vi "Pedestal_viewer (Module).vi"(0 "ACQ full DATA file path":path caption="File path", 5 "ChipID list":u32[](array[numeric]) format="%.0x", 7 "quants events per chip":u32[](array[numeric]), 9 "ID summary":string, 11 "ACQ events fets":u32=80 caption="Acquired events") -> ()   [LabVIEW 2015, in "VIPM2.lvlib"]
doc: "<b>Acquisition Data viewer</b>\nInclou ACQ choose Chip Data_viewer.vi"
uses:
  VIPM2.lvlib
  <vilib>/Analysis/NI_AALBase.lvlib
panel:
  out "Barra Load events":i32(slide) scale=-1.0..3600000.0
  in  "X scale max.":dbl=150.0 min=0.0 max=1e+29 step=10.0
  in  "X scale min.":dbl=80.0 min=0.0 max=1e+29 step=10.0
  in  "Y scale":dbl=100.0 min=5.0 max=1e+29 step=10.0
  in  "Take image button":bool
  in  "Choose Chip button":bool
  in  "Close button":bool
  out "Total number of events":u32 caption="Total number of events\nCentrals + Neighbors"
  out "data time":string
  out "Chip ID":string
  out "Trigger histogram 99":T1(graph)
  out "Trigger histogram 98":T1(graph)
  out "Trigger histogram 97":T1(graph)
  out "Trigger histogram 96":T1(graph)
  out "Trigger histogram 95":T1(graph)
  out "Trigger histogram 94":T1(graph)
  out "Trigger histogram 93":T1(graph)
  out "Trigger histogram 92":T1(graph)
  out "Trigger histogram 91":T1(graph)
  out "Trigger histogram 90":T1(graph)
  out "Trigger histogram 89":T1(graph)
  out "Trigger histogram 88":T1(graph)
  out "Trigger histogram 87":T1(graph)
  out "Trigger histogram 86":T1(graph)
  out "Trigger histogram 85":T1(graph)
  out "Trigger histogram 84":T1(graph)
  out "Trigger histogram 83":T1(graph)
  out "Trigger histogram 82":T1(graph)
  out "Trigger histogram 81":T1(graph)
  out "Trigger histogram 80":T1(graph)
  out "Trigger histogram 79":T1(graph)
  out "Trigger histogram 78":T1(graph)
  out "Trigger histogram 77":T1(graph)
  out "Trigger histogram 76":T1(graph)
  out "Trigger histogram 75":T1(graph)
  out "Trigger histogram 74":T1(graph)
  out "Trigger histogram 73":T1(graph)
  out "Trigger histogram 72":T1(graph)
  out "Trigger histogram 71":T1(graph)
  out "Trigger histogram 70":T1(graph)
  out "Trigger histogram 69":T1(graph)
  out "Trigger histogram 68":T1(graph)
  out "Trigger histogram 67":T1(graph)
  out "Trigger histogram 66":T1(graph)
  out "Trigger histogram 65":T1(graph)
  out "Trigger histogram 64":T1(graph)
  out "Trigger histogram 63":T1(graph)
  out "Trigger histogram 62":T1(graph)
  out "Trigger histogram 61":T1(graph)
  out "Trigger histogram 60":T1(graph)
  out "Trigger histogram 59":T1(graph)
  out "Trigger histogram 58":T1(graph)
  out "Trigger histogram 57":T1(graph)
  out "Trigger histogram 56":T1(graph)
  out "Trigger histogram 55":T1(graph)
  out "Trigger histogram 54":T1(graph)
  out "Trigger histogram 53":T1(graph)
  out "Trigger histogram 52":T1(graph)
  out "Trigger histogram 51":T1(graph)
  out "Trigger histogram 50":T1(graph)
  out "Trigger histogram 49":T1(graph)
  out "Trigger histogram 48":T1(graph)
  out "Trigger histogram 47":T1(graph)
  out "Trigger histogram 46":T1(graph)
  out "Trigger histogram 45":T1(graph)
  out "Trigger histogram 44":T1(graph)
  out "Trigger histogram 43":T1(graph)
  out "Trigger histogram 42":T1(graph)
  out "Trigger histogram 41":T1(graph)
  out "Trigger histogram 40":T1(graph)
  out "Trigger histogram 39":T1(graph)
  out "Trigger histogram 38":T1(graph)
  out "Trigger histogram 37":T1(graph)
  out "Trigger histogram 36":T1(graph)
  out "Trigger histogram 35":T1(graph)
  out "Trigger histogram 34":T1(graph)
  out "Trigger histogram 33":T1(graph)
  out "Trigger histogram 32":T1(graph)
  out "Trigger histogram 31":T1(graph)
  out "Trigger histogram 30":T1(graph)
  out "Trigger histogram 29":T1(graph)
  out "Trigger histogram 28":T1(graph)
  out "Trigger histogram 27":T1(graph)
  out "Trigger histogram 26":T1(graph)
  out "Trigger histogram 25":T1(graph)
  out "Trigger histogram 24":T1(graph)
  out "Trigger histogram 23":T1(graph)
  out "Trigger histogram 22":T1(graph)
  out "Trigger histogram 21":T1(graph)
  out "Trigger histogram 20":T1(graph)
  out "Trigger histogram 19":T1(graph)
  out "Trigger histogram 18":T1(graph)
  out "Trigger histogram 17":T1(graph)
  out "Trigger histogram 16":T1(graph)
  out "Trigger histogram 15":T1(graph)
  out "Trigger histogram 14":T1(graph)
  out "Trigger histogram 13":T1(graph)
  out "Trigger histogram 12":T1(graph)
  out "Trigger histogram 11":T1(graph)
  out "Trigger histogram 10":T1(graph)
  out "Trigger histogram 09":T1(graph)
  out "Trigger histogram 08":T1(graph)
  out "Trigger histogram 07":T1(graph)
  out "Trigger histogram 06":T1(graph)
  out "Trigger histogram 05":T1(graph)
  out "Trigger histogram 04":T1(graph)
  out "Trigger histogram 03":T1(graph)
  out "Trigger histogram 01":T1(graph)
  out "Trigger histogram 00":T1(graph)
  out "Trigger histogram 02":T1(graph)
  out "100px Trigger Data":cluster{"1px Trigger Data":u16[]}[](array[cluster])
  # "99"
  # "98"
  # "97"
  # "96"
  # "95"
  # "94"
  # "93"
  # "92"
  # "91"
  # "90"
  # "89"
  # "88"
  # "87"
  # "86"
  # "85"
  # "84"
  # "83"
  # "82"
  # "81"
  # "80"
  # "79"
  # "78"
  # "77"
  # "76"
  # "75"
  # "74"
  # "73"
  # "72"
  # "71"
  # "70"
  # "69"
  # "68"
  # "67"
  # "66"
  # "65"
  # "64"
  # "63"
  # "62"
  # "61"
  # "60"
  # "59"
  # "58"
  # "57"
  # "56"
  # "55"
  # "54"
  # "53"
  # "52"
  # "51"
  # "50"
  # "49"
  # "48"
  # "47"
  # "46"
  # "45"
  # "44"
  # "43"
  # "42"
  # "41"
  # "40"
  # "39"
  # "38"
  # "37"
  # "36"
  # "35"
  # "34"
  # "33"
  # "32"
  # "31"
  # "30"
  # "29"
  # "28"
  # "27"
  # "26"
  # "25"
  # "24"
  # "23"
  # "22"
  # "21"
  # "20"
  # "19"
  # "18"
  # "17"
  # "16"
  # "15"
  # "14"
  # "13"
  # "12"
  # "11"
  # "10"
  # "09"
  # "08"
  # "07"
  # "06"
  # "05"
  # "04"
  # "03"
  # "01"
  # "00"
  # "02"
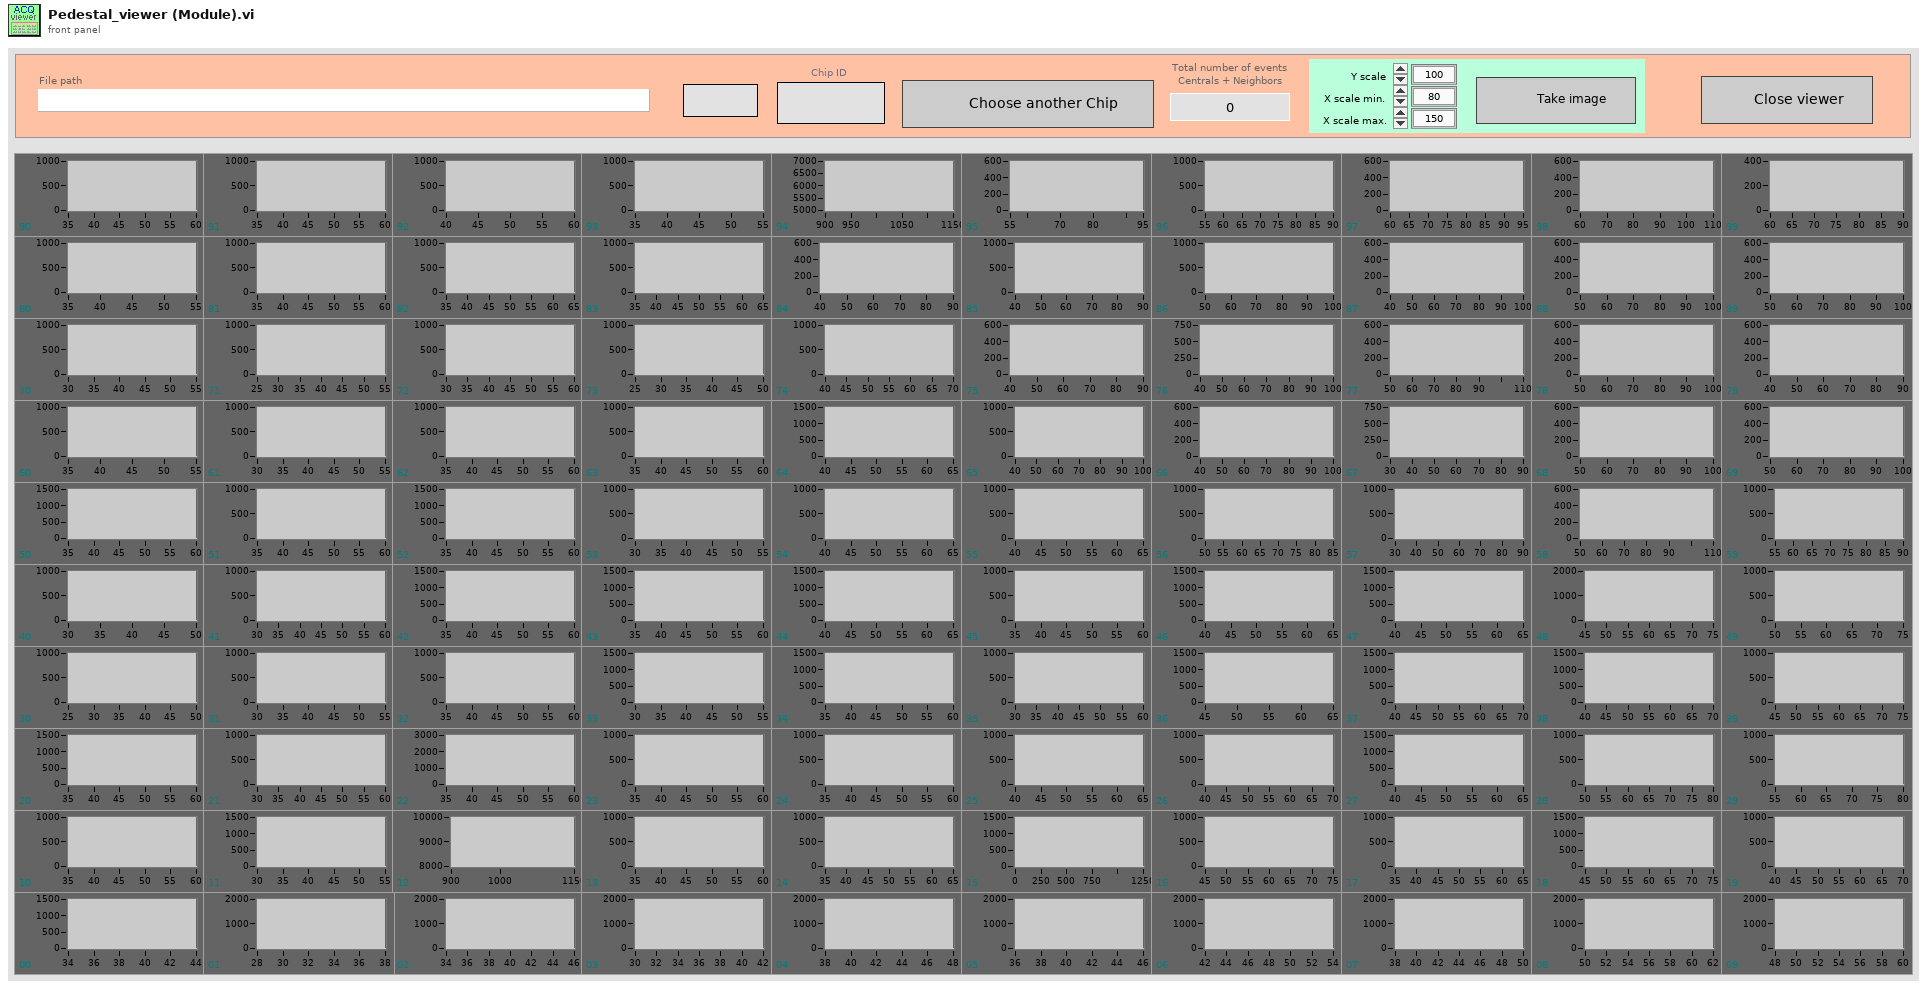
[diagram p1: front panel]
types:
  T1 = cluster{"X Values":dbl[], "Histogram: h(x)":i32[]}
  T2 = enum16{"big-endian, network order", "native, host order", "little-endian"}
  T3 = typedef "imagedata.ctl" = cluster{"image type":i32, "image depth":i32, "image":u8[], "mask":u8[], "colors":u32[], "Rectangle":cluster{"left":i16, "top":i16, "right":i16, "bottom":i16}}
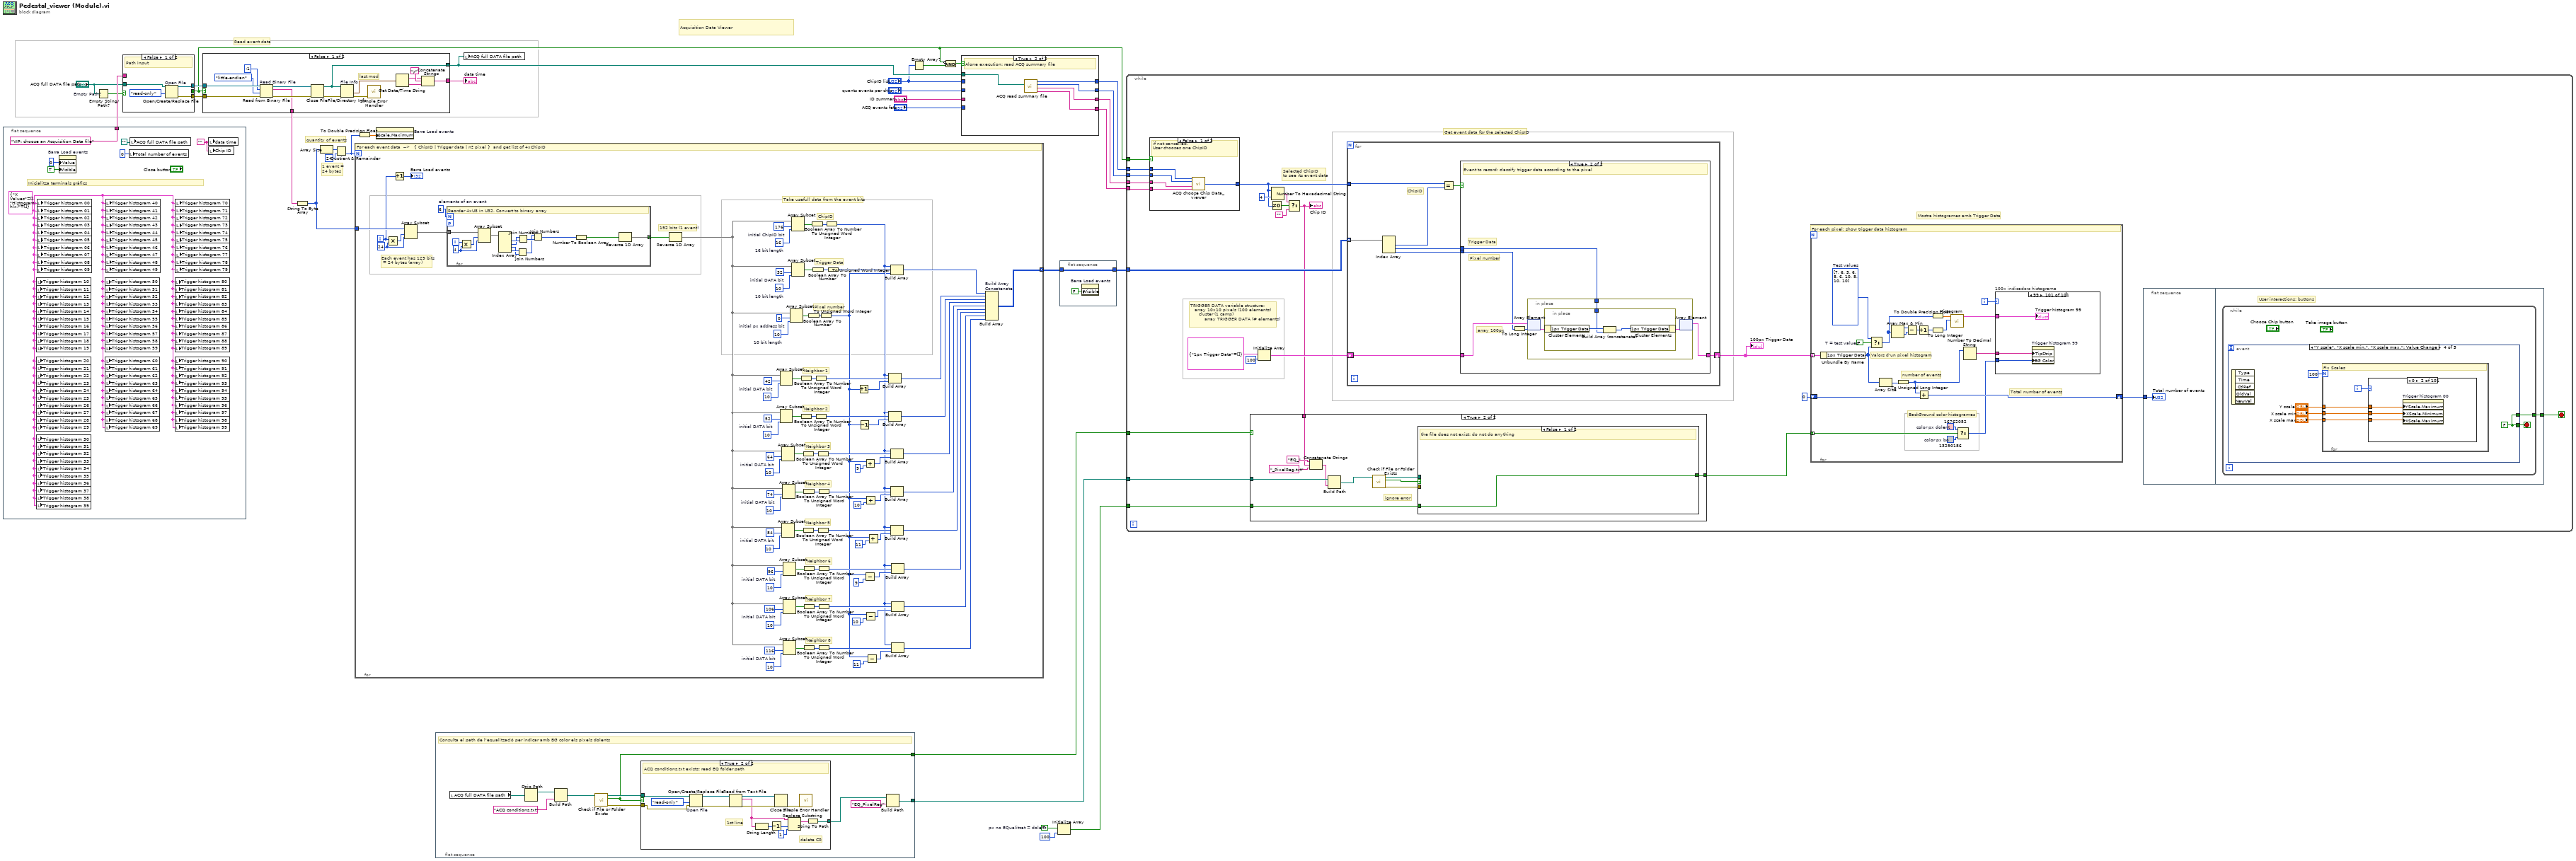
[diagram p0: block diagram]
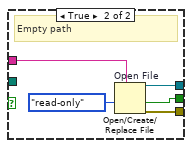
[diagram p3: hidden frame]
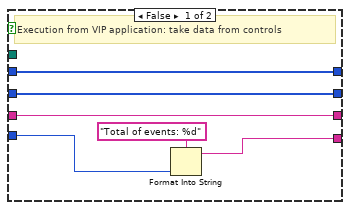
[diagram p5: hidden frame]
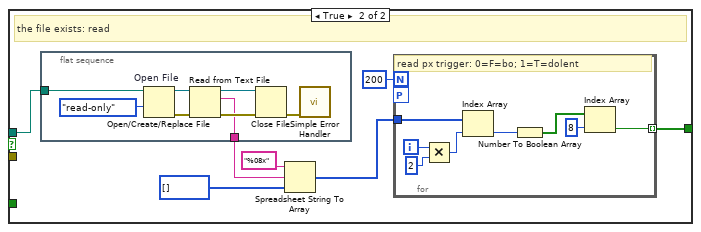
[diagram p7: hidden frame]
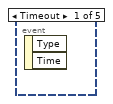
[diagram p9: hidden frame]
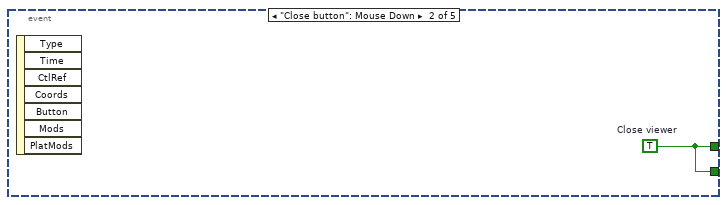
[diagram p10: hidden frame]
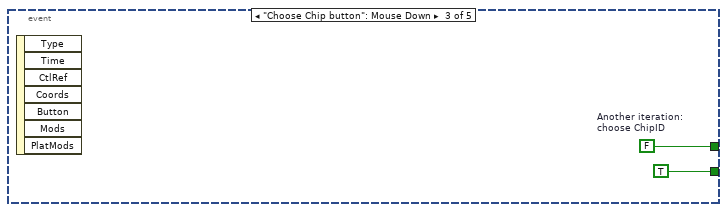
[diagram p11: hidden frame]
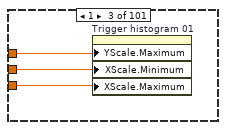
[diagram p13: hidden frame]
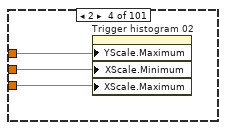
[diagram p14: hidden frame]
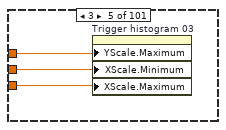
[diagram p15: hidden frame]
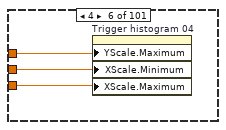
[diagram p16: hidden frame]
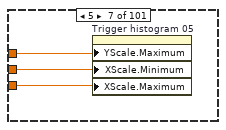
[diagram p17: hidden frame]
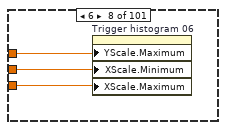
[diagram p18: hidden frame]
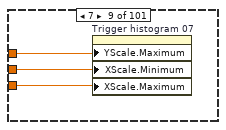
[diagram p19: hidden frame]
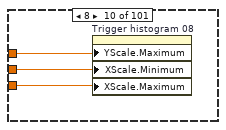
[diagram p20: hidden frame]
diagram:
  w2 = TRUE  # px no EQualitzat = dolent
  # "1 event =\n24 bytes"
  # "quantity of events"
  # "Read event data"
  # "Acquisition Data Viewer"
  n1 = flat-sequence {
    tunnel: ["VIP: choose an Acquisition Data file" ("prompt")] -> w28
    frame #0 {
      w34 = T1 {"X Values"=[], "Histogram: h(x)"=[]} ("Trigger histogram 00")
      w36 = ""
      # "Inicialitza terminals gràfics"
      n2 = local write "Trigger histogram 10"(w34) -> ()
      n3 = local write "Trigger histogram 11"(w34) -> ()
      n4 = local write "Trigger histogram 12"(w34) -> ()
      n5 = local write "Trigger histogram 13"(w34) -> ()
      n6 = local write "Trigger histogram 14"(w34) -> ()
      n7 = local write "Trigger histogram 15"(w34) -> ()
      n8 = local write "Trigger histogram 16"(w34) -> ()
      n9 = local write "Trigger histogram 17"(w34) -> ()
      n10 = local write "Trigger histogram 18"(w34) -> ()
      n11 = local write "Trigger histogram 19"(w34) -> ()
      n12 = local write "Trigger histogram 20"(w34) -> ()
      n13 = local write "Trigger histogram 21"(w34) -> ()
      n14 = local write "Trigger histogram 22"(w34) -> ()
      n15 = local write "Trigger histogram 23"(w34) -> ()
      n16 = local write "Trigger histogram 24"(w34) -> ()
      n17 = local write "Trigger histogram 25"(w34) -> ()
      n18 = local write "Trigger histogram 26"(w34) -> ()
      n19 = local write "Trigger histogram 27"(w34) -> ()
      n20 = local write "Trigger histogram 28"(w34) -> ()
      n21 = local write "Trigger histogram 29"(w34) -> ()
      n22 = local write "Trigger histogram 30"(w34) -> ()
      n23 = local write "Trigger histogram 31"(w34) -> ()
      n24 = local write "Trigger histogram 32"(w34) -> ()
      n25 = local write "Trigger histogram 33"(w34) -> ()
      n26 = local write "Trigger histogram 34"(w34) -> ()
      n27 = local write "Trigger histogram 35"(w34) -> ()
      n28 = local write "Trigger histogram 36"(w34) -> ()
      n29 = local write "Trigger histogram 37"(w34) -> ()
      n30 = local write "Trigger histogram 38"(w34) -> ()
      n31 = local write "Trigger histogram 39"(w34) -> ()
      n32 = local write "Trigger histogram 00"(w34) -> ()
      n33 = local write "Trigger histogram 01"(w34) -> ()
      n34 = local write "Trigger histogram 02"(w34) -> ()
      n35 = local write "Trigger histogram 03"(w34) -> ()
      n36 = local write "Trigger histogram 04"(w34) -> ()
      n37 = local write "Trigger histogram 05"(w34) -> ()
      n38 = local write "Trigger histogram 06"(w34) -> ()
      n39 = local write "Trigger histogram 07"(w34) -> ()
      n40 = local write "Trigger histogram 08"(w34) -> ()
      n41 = local write "Trigger histogram 09"(w34) -> ()
      n42 = property on="Barra Load events" class="Slide (strict)"("Value"=0 ("Barra Load events"), "Visible"=TRUE) -> ()  [unwired: 2 in, 2 out]
      n43 = local write "Trigger histogram 50"(w34) -> ()
      n44 = local write "Trigger histogram 51"(w34) -> ()
      n45 = local write "Trigger histogram 52"(w34) -> ()
      n46 = local write "Trigger histogram 53"(w34) -> ()
      n47 = local write "Trigger histogram 54"(w34) -> ()
      n48 = local write "Trigger histogram 55"(w34) -> ()
      n49 = local write "Trigger histogram 56"(w34) -> ()
      n50 = local write "Trigger histogram 57"(w34) -> ()
      n51 = local write "Trigger histogram 58"(w34) -> ()
      n52 = local write "Trigger histogram 59"(w34) -> ()
      n53 = local write "Trigger histogram 60"(w34) -> ()
      n54 = local write "Trigger histogram 61"(w34) -> ()
      n55 = local write "Trigger histogram 62"(w34) -> ()
      n56 = local write "Trigger histogram 63"(w34) -> ()
      n57 = local write "Trigger histogram 64"(w34) -> ()
      n58 = local write "Trigger histogram 65"(w34) -> ()
      n59 = local write "Trigger histogram 66"(w34) -> ()
      n60 = local write "Trigger histogram 67"(w34) -> ()
      n61 = local write "Trigger histogram 68"(w34) -> ()
      n62 = local write "Trigger histogram 69"(w34) -> ()
      n63 = local write "Trigger histogram 40"(w34) -> ()
      n64 = local write "Trigger histogram 41"(w34) -> ()
      n65 = local write "Trigger histogram 42"(w34) -> ()
      n66 = local write "Trigger histogram 43"(w34) -> ()
      n67 = local write "Trigger histogram 44"(w34) -> ()
      n68 = local write "Trigger histogram 45"(w34) -> ()
      n69 = local write "Trigger histogram 46"(w34) -> ()
      n70 = local write "Trigger histogram 47"(w34) -> ()
      n71 = local write "Trigger histogram 48"(w34) -> ()
      n72 = local write "Trigger histogram 49"(w34) -> ()
      n73 = local write "Total number of events"(u32 0 ("Total number of events")) -> ()
      n74 = local write "ACQ full DATA file path"(path "") -> ()
      n75 = local write "Trigger histogram 80"(w34) -> ()
      n76 = local write "Trigger histogram 81"(w34) -> ()
      n77 = local write "Trigger histogram 82"(w34) -> ()
      n78 = local write "Trigger histogram 83"(w34) -> ()
      n79 = local write "Trigger histogram 84"(w34) -> ()
      n80 = local write "Trigger histogram 85"(w34) -> ()
      n81 = local write "Trigger histogram 86"(w34) -> ()
      n82 = local write "Trigger histogram 87"(w34) -> ()
      n83 = local write "Trigger histogram 88"(w34) -> ()
      n84 = local write "Trigger histogram 89"(w34) -> ()
      n85 = local write "Trigger histogram 90"(w34) -> ()
      n86 = local write "Trigger histogram 91"(w34) -> ()
      n87 = local write "Trigger histogram 92"(w34) -> ()
      n88 = local write "Trigger histogram 93"(w34) -> ()
      n89 = local write "Trigger histogram 94"(w34) -> ()
      n90 = local write "Trigger histogram 95"(w34) -> ()
      n91 = local write "Trigger histogram 96"(w34) -> ()
      n92 = local write "Trigger histogram 97"(w34) -> ()
      n93 = local write "Trigger histogram 98"(w34) -> ()
      n94 = local write "Trigger histogram 99"(w34) -> ()
      n95 = local write "Trigger histogram 70"(w34) -> ()
      n96 = local write "Trigger histogram 71"(w34) -> ()
      n97 = local write "Trigger histogram 72"(w34) -> ()
      n98 = local write "Trigger histogram 73"(w34) -> ()
      n99 = local write "Trigger histogram 74"(w34) -> ()
      n100 = local write "Trigger histogram 75"(w34) -> ()
      n101 = local write "Trigger histogram 76"(w34) -> ()
      n102 = local write "Trigger histogram 77"(w34) -> ()
      n103 = local write "Trigger histogram 78"(w34) -> ()
      n104 = local write "Trigger histogram 79"(w34) -> ()
      n105 = local write "data time"(w36) -> ()
      n106 = local write "Chip ID"(w36) -> ()
    }
  }
  n107 = Empty String/Path? "Empty Path?"(string/path="ACQ full DATA file path") -> (empty?=w27:bool)
  n108 = case shown="False" w27 {
    tunnel: [w41 w46] -> w31
    tunnel: [w40 w45] -> w30
    tunnel: [_ w44] -> w7
    tunnel: w28 -> [_ w43]
    tunnel: "ACQ full DATA file path" -> [w39 _]
    frame False {
      # "Path input"
      n109 = Open/Create/Replace File "Open File"(file path (use dialog)=w39, access (0:read/write)=enum16{"read/write", "read-only", "write-only"}."read-only") -> (refnum out=w40:refnum<file>, error out=w41:errorcluster)  [unwired: 4 in, 1 out]
    }
    frame True {
      # "Empty path"
      n110 = Open/Create/Replace File "Open File"(prompt=w43, access (0:read/write)=enum16{"read/write", "read-only", "write-only"}."read-only") -> (refnum out=w45:refnum<file>, cancelled=w44:bool, error out=w46:errorcluster)  [unwired: 4 in]
    }
  }
  n111 = case shown="False" w7 {
    tunnel: w31 -> [w62 _]
    tunnel: w30 -> [w61 _]
    tunnel: [w56 _] -> w23
    tunnel: [w49 _] -> w29
    tunnel: [w48 _] -> w18
    frame False {
      # "last mod"
      n112 = Read from Binary File "Read Binary File"(8:w62, 9:T2."little-endian" ("byte order (0:big-endian, network order)"), 10:-1 ("count (1)"), 11:w61) -> (0:w59:errorcluster, 2:w56:string, 3:w58:refnum<file>)  [unwired: 2 in, 1 out]
      n113 = Close File(refnum=w58, error in=w59) -> (path=w48:path, error out=w55:errorcluster)
      n114 = File/Directory Info "File Info"(path=w48, error in=w55) -> (last mod=w50:timestamp, error out=w54:errorcluster)  [unwired: 5 out]
      n115 = call <vilib>:"Simple Error Handler.vi"("error in (no error)"=w54) -> ()  [unwired: 4 in, 5 out]
      n116 = Get Date/Time String(seconds (now)=w50) -> (date string=w51:string, time string=w53:string)  [unwired: 2 in]
      n117 = Concatenate Strings(w51, "\r", w53) -> (w49:string)
    }
    frame True {
      # "Openning cancelled"
    }
  }
  "data time" <- w29
  n118 = String To Byte Array(string=w23) -> (unsigned byte array=w6:u8[])
  n119 = Array Size(array=w6) -> (size(s)=w24:i32)
  n120 = Quotient & Remainder(x=w24, y=24) -> (floor(x/y)=w21:i32)  [unwired: 1 out]
  n121 = for {
    N: w21 -> [_]
    tunnel: w6 -> [w146]
    tunnel: [w128] -> w19 mode=concatenating
    i -> [w130]
    w89 = 116  # initial DATA bit
    w94 = 106  # initial DATA bit
    w99 = 96  # initial DATA bit
    w104 = 84  # initial DATA bit
    w109 = 74  # initial DATA bit
    w114 = 64  # initial DATA bit
    w119 = 52  # initial DATA bit
    w126 = 42  # initial DATA bit
    w135 = 10  # 10 bit length
    w136 = 0  # initial px address bit
    w140 = 10  # 10 bit length
    w139 = 32  # initial DATA bit
    w143 = 16  # 16 bit length
    w144 = 176  # initial ChipID bit
    w149 = 24 ("y")
    w150 = 6  # elements of an event
    # "Neighbor 8"
    # "Neighbor 7"
    # "Neighbor 6"
    # "Neighbor 5"
    # "Neighbor 4"
    # "Neighbor 3"
    # "Neighbor 2"
    # "Neighbor 1"
    # "Take usefull data from the event bits"
    # "Pixel number"
    # "Trigger Data"
    # "ChipID"
    # "192 bits (1 event)"
    # "Each event has 129 bits\n = 24 bytes (array)"
    # "For each event data  -->   { ChipID | Trigger data | nº pixel }  and get list of 4xChipID"
    n122 = Multiply(x=w130, y=w149) -> (x*y=w148:i32)
    n123 = Increment(x=w130) -> (x+1=→"Barra Load events":i32)
    n124 = Array Subset "Array Subset"(array=w146, index=w148, length=w149) -> (w147:u8[])
    n125 = for {
      N: w150 -> [_]
      tunnel: w147 -> [w163]
      workers-P: _ -> [_]
      tunnel: [w151] -> w145 mode=concatenating
      i -> [w164]
      w161 = 4 ("y")
      # "Reorder 4xU8 in U32. Convert to binary array"
      n126 = Multiply(x=w164, y=w161) -> (x*y=w162:i32)
      n127 = Array Subset "Array Subset"(array=w163, index=w162, length=w161) -> (w160:u8[])
      n128 = Index Array(array=w160) -> (element #1=w159:u8, element #2=w158:u8, element #3=w156:u8, element #4=w157:u8)  [unwired: 4 in]
      n129 = Join Numbers(hi=w157, lo=w156) -> ((hi.lo)=w154:u16)
      n130 = Join Numbers(hi=w158, lo=w159) -> ((hi.lo)=w155:u16)
      n131 = Join Numbers(hi=w154, lo=w155) -> ((hi.lo)=w152:u32)
      n132 = Number To Boolean Array(number=w152) -> (Boolean array=w153:bool[])
      n133 = Reverse 1D Array(array=w153) -> (reversed array=w151:bool[])
    }
    n134 = Reverse 1D Array(array=w145) -> (reversed array=w68:bool[])
    n135 = Array Subset "Array Subset"(array=w68, index=w126, length=10 ("10 bit length")) -> (w124:bool[])
    n136 = Array Subset "Array Subset"(array=w68, index=w119, length=10 ("10 bit length")) -> (w117:bool[])
    n137 = Array Subset "Array Subset"(array=w68, index=w114, length=10 ("10 bit length")) -> (w112:bool[])
    n138 = Array Subset "Array Subset"(array=w68, index=w104, length=10 ("10 bit length")) -> (w102:bool[])
    n139 = Array Subset "Array Subset"(array=w68, index=w109, length=10 ("10 bit length")) -> (w107:bool[])
    n140 = Array Subset "Array Subset"(array=w68, index=w99, length=10 ("10 bit length")) -> (w97:bool[])
    n141 = Array Subset "Array Subset"(array=w68, index=w94, length=10 ("10 bit length")) -> (w92:bool[])
    n142 = Array Subset "Array Subset"(array=w68, index=w89, length=10 ("10 bit length")) -> (w87:bool[])
    n143 = Array Subset "Array Subset"(array=w68, index=w136, length=w135) -> (w134:bool[])
    n144 = Array Subset "Array Subset"(array=w68, index=w144, length=w143) -> (w142:bool[])
    n145 = Array Subset "Array Subset"(array=w68, index=w139, length=w140) -> (w137:bool[])
    n146 = Boolean Array To Number(Boolean array=w124) -> (number=w125:u32)
    n147 = Boolean Array To Number(Boolean array=w117) -> (number=w118:u32)
    n148 = Boolean Array To Number(Boolean array=w112) -> (number=w113:u32)
    n149 = Boolean Array To Number(Boolean array=w102) -> (number=w103:u32)
    n150 = Boolean Array To Number(Boolean array=w107) -> (number=w108:u32)
    n151 = Boolean Array To Number(Boolean array=w97) -> (number=w98:u32)
    n152 = Boolean Array To Number(Boolean array=w92) -> (number=w93:u32)
    n153 = Boolean Array To Number(Boolean array=w87) -> (number=w88:u32)
    n154 = Boolean Array To Number(Boolean array=w134) -> (number=w133:u32)
    n155 = Boolean Array To Number(Boolean array=w142) -> (number=w141:u32)
    n156 = Boolean Array To Number(Boolean array=w137) -> (number=w138:u32)
    n157 = To Unsigned Word Integer(number=w125) -> (unsigned 16bit integer=w123:u16)
    n158 = To Unsigned Word Integer(number=w118) -> (unsigned 16bit integer=w116:u16)
    n159 = To Unsigned Word Integer(number=w113) -> (unsigned 16bit integer=w111:u16)
    n160 = To Unsigned Word Integer(number=w103) -> (unsigned 16bit integer=w101:u16)
    n161 = To Unsigned Word Integer(number=w108) -> (unsigned 16bit integer=w106:u16)
    n162 = To Unsigned Word Integer(number=w98) -> (unsigned 16bit integer=w96:u16)
    n163 = To Unsigned Word Integer(number=w93) -> (unsigned 16bit integer=w91:u16)
    n164 = To Unsigned Word Integer(number=w88) -> (unsigned 16bit integer=w86:u16)
    n165 = To Unsigned Word Integer(number=w133) -> (unsigned 16bit integer=w66:u16)
    n166 = To Unsigned Word Integer(number=w141) -> (unsigned 16bit integer=w67:u16)
    n167 = To Unsigned Word Integer(number=w138) -> (unsigned 16bit integer=w132:u16)
    n168 = Increment(x=w66) -> (x+1=w122:u16)
    n169 = Decrement(x=w66) -> (x-1=w85:u16)
    n170 = Subtract(x=w66, y=u16 9) -> (x-y=w73:u16)
    n171 = Add(x=w66, y=u16 9) -> (x+y=w82:u16)
    n172 = Add(x=w66, y=u16 10) -> (x+y=w79:u16)
    n173 = Subtract(x=w66, y=u16 10) -> (x-y=w70:u16)
    n174 = Subtract(x=w66, y=u16 11) -> (x-y=w64:u16)
    n175 = Add(x=w66, y=u16 11) -> (x+y=w76:u16)
    n176 = Build Array "Build Array"(w67, w123, w122) -> (w121:u16[])
    n177 = Build Array "Build Array"(w67, w116, w85) -> (w84:u16[])
    n178 = Build Array "Build Array"(w67, w111, w82) -> (w81:u16[])
    n179 = Build Array "Build Array"(w67, w101, w76) -> (w75:u16[])
    n180 = Build Array "Build Array"(w67, w132, w66) -> (w129:u16[])
    n181 = Build Array "Build Array"(w67, w106, w79) -> (w78:u16[])
    n182 = Build Array "Build Array"(w67, w96, w73) -> (w72:u16[])
    n183 = Build Array "Build Array"(w67, w91, w70) -> (w69:u16[])
    n184 = Build Array "Build Array"(w67, w86, w64) -> (w63:u16[])
    n185 = Build Array "Build Array\nConcatenate"(w129, w121, w84, w81, w78, w75, w72, w69, w63) -> (w128:u16[][])
  }
  n186 = To Double Precision Float(number=w21) -> (double precision float=w22:dbl)
  n187 = property on="Barra Load events" class="Slide (strict)"("Scale.Maximum"=w22) -> ()  [unwired: 2 in, 2 out]
  n188 = flat-sequence {
    tunnel: [w165] -> w4
    tunnel: [w168] -> w5
    frame #0 {
      # "Consulta el path de l'equalització per indicar amb BG color els pixels dolents"
      n189 = local read "ACQ full DATA file path"() -> (w169:path)
      n190 = Strip Path(path=w169) -> (stripped path=w170:path)  [unwired: 1 out]
      n191 = Build Path(base path=w170, name or relative path="ACQ conditions.txt") -> (appended path=w172:path)
      n192 = call <vilib>:"Check if File or Folder Exists.vi"("path"=w172) -> ("error out"=w174:errorcluster, "file or folder exists?"=w168:bool, "dup path"=w173:path)  [unwired: 8 in]
      n193 = case shown="True" w168 {
        tunnel: w173 -> [_ w188]
        tunnel: w174 -> [_ w186]
        tunnel: [_ w175] -> w166
        frame False {
          # "ACQ conditions.txt doesn't exist"
        }
        frame True {
          # "delete CR"
          # "1st line"
          # "ACQ conditions.txt exists: read EQ folder path"
          n194 = Open/Create/Replace File "Open File"(file path (use dialog)=w188, error in=w186, access (0:read/write)=enum16{"read/write", "read-only", "write-only"}."read-only") -> (refnum out=w185:refnum<file>, error out=w184:errorcluster)  [unwired: 3 in, 1 out]
          n195 = Read from Text File(file (use dialog)=w185, error in=w184) -> (refnum out=w183:refnum<file>, text=w176:string, error out=w182:errorcluster)  [unwired: 2 in, 1 out]
          n196 = String Length(string=w176) -> (length=w180:i32)
          n197 = Decrement(x=w180) -> (x-1=w179:i32)
          n198 = Close File(refnum=w183, error in=w182) -> (error out=w181:errorcluster)  [unwired: 1 out]
          n199 = Replace Substring(2:1 ("length (len. of substring)"), 3:w179, 5:w176) -> (1:w177:string)  [unwired: 1 in, 1 out]
          n200 = call <vilib>:"Simple Error Handler.vi"("error in (no error)"=w181) -> ()  [unwired: 4 in, 5 out]
          n201 = String To Path(string=w177) -> (path=w175:path)
        }
      }
      n202 = Build Path(base path=w166, name or relative path="EQ_PixelReg") -> (appended path=w165:path)
    }
  }
  n203 = local write "ACQ full DATA file path"(w18) -> ()
  n204 = Empty Array?(array="ChipID list") -> (empty?=w9:bool)
  n205 = Compound Arithmetic op=AND(invert w7, w9) -> (w8:bool)
  n206 = case shown="True" w8 {
    tunnel: w18 -> [_ w199]
    tunnel: "ChipID list" -> [w194 _]
    tunnel: [w194 w198] -> w10
    tunnel: [w193 w197] -> w11
    tunnel: "quants events per chip" -> [w193 _]
    tunnel: "ID summary" -> [w192 _]
    tunnel: "ACQ events fets" -> [w190 _]
    tunnel: [w192 w196] -> w12
    tunnel: [w189 w195] -> w13
    frame False {
      # "Execution from VIP application: take data from controls"
      n207 = Format Into String "Format Into String"(format string="Total of events: %d", w190) -> (resulting string=w189:string)  [unwired: 2 in, 1 out]
    }
    frame True {
      # "Alone execution: read ACQ summary file"
      n208 = call "ACQ read summary file.vi"("ACQ binary data file path"=w199) -> ("Total of events"=w195:string, "ID summary"=w196:string, "quants events per chip"=w197:u32[], "ChipID list"=w198:u32[])  [unwired: 7 in]
    }
  }
  n209 = Initialize Array "Initialize Array"(w2, 100 ("dimension size")) -> (w1:bool[])
  n210 = flat-sequence {
    tunnel: [w201] -> w20
    tunnel: w19 -> [w201]
    frame #0 {
      n211 = property on="Barra Load events" class="Slide (strict)"("Visible"=FALSE) -> ()  [unwired: 2 in, 2 out]
    }
  }
  n212 = while {
    tunnel: w20 -> [w224]
    tunnel: w13 -> [w211]
    tunnel: w12 -> [w210]
    tunnel: w11 -> [w209]
    tunnel: w10 -> [w208]
    tunnel: w7 -> [w207]
    tunnel: w5 -> [w205]
    tunnel: w4 -> [w204]
    tunnel: w1 -> [w203]
    stop <- w218 stop-if-true
    # "Mostra histogrames amb Trigger Data"
    # "TRIGGER DATA variable structure:\n   array 10x10 pixels (100 elements)\n      cluster (1 camp)\n          array TRIGGER DATA (# elements)"
    # "Get event data for the selected ChipID"
    # "Selected ChipID\nto see its event data"
    n213 = case shown="False" w207 {
      tunnel: [w265 _] -> w212
      tunnel: w211 -> [w264 _]
      tunnel: w210 -> [w263 _]
      tunnel: w209 -> [w262 _]
      tunnel: w208 -> [w261 _]
      frame False {
        # "if not cancelled,\nUser chooses one ChipID"
        n214 = call "ACQ choose Chip Data_viewer.vi"("Chip ID list"=w261, "quants events per Chip"=w262, "summary IDs"=w263, "Total of events"=w264) -> ("ChipID choosed"=w265:u16)  [unwired: 11 in]
      }
      frame True {
      }
    }
    n215 = Initialize Array "Initialize Array"(cluster{"1px Trigger Data":u16[]} {"1px Trigger Data"=[]} ("1px Trigger Data"), 100 ("dimension size")) -> (w221:cluster{"1px Trigger Data":u16[]}[])
    n216 = Not Equal To 0?(x=w212) -> (x != 0?=w215:bool)
    n217 = Number To Hexadecimal String(1:i16 4 ("width (-)"), 2:w212) -> (0:w216:string)
    n218 = Select(t=w216, s=w215, f="") -> (s? t:f=w206:string)
    "Chip ID" <- w206
    n219 = case shown="True" w205 {
      tunnel: w204 -> [_ w236]
      tunnel: w206 -> [_ w234]
      tunnel: [w225 w227] -> w202
      tunnel: w203 -> [w225 w226]
      frame False {
      }
      frame True {
        # "ignore error"
        n220 = Concatenate Strings "Concatenate Strings"("EQ_", w234, "_PixelReg.txt") -> (w232:string)
        n221 = Build Path(base path=w236, name or relative path=w232) -> (appended path=w231:path)
        n222 = call <vilib>:"Check if File or Folder Exists.vi"("path"=w231) -> ("error out"=w228:errorcluster, "file or folder exists?"=w229:bool, "dup path"=w230:path)  [unwired: 8 in]
        n223 = case shown="False" w229 {
          tunnel: w230 -> [_ w244]
          tunnel: w228 -> [_ _]
          tunnel: [w237 w238] -> w227
          tunnel: w226 -> [w237 _]
          frame False {
            # "the file does not exist: do not do anything"
          }
          frame True {
            # "the file exists: read"
            n224 = flat-sequence {
              tunnel: w244 -> [w260]
              tunnel: [w253] -> w243
              frame #0 {
                n225 = Open/Create/Replace File "Open File"(file path (use dialog)=w260, access (0:read/write)=enum16{"read/write", "read-only", "write-only"}."read-only") -> (refnum out=w257:refnum<file>, error out=w258:errorcluster)  [unwired: 4 in, 1 out]
                n226 = Read from Text File(file (use dialog)=w257, error in=w258) -> (refnum out=w256:refnum<file>, text=w253:string, error out=w255:errorcluster)  [unwired: 2 in, 1 out]
                n227 = Close File(refnum=w256, error in=w255) -> (error out=w254:errorcluster)  [unwired: 1 out]
                n228 = call <vilib>:"Simple Error Handler.vi"("error in (no error)"=w254) -> ()  [unwired: 4 in, 5 out]
              }
            }
            n229 = Spreadsheet String To Array(format string="%08x", spreadsheet string=w243, array type (2D Dbl)=u32[] []) -> (array=w240:u32[])  [unwired: 1 in]
            n230 = for {
              N: 200 -> [_]
              tunnel: w240 -> [w249]
              tunnel: [w245] -> w238 mode=indexing
              workers-P: _ -> [_]
              i -> [w252]
              # "read px trigger: 0=F=bo; 1=T=dolent"
              n231 = Multiply(x=w252, y=2) -> (x*y=w250:i32)
              n232 = Index Array "Index Array"(array=w249, index=w250) -> (element=w248:u32)
              n233 = Number To Boolean Array(number=w248) -> (Boolean array=w247:bool[])
              n234 = Index Array "Index Array"(array=w247, index=8) -> (element=w245:bool)
            }
          }
        }
      }
    }
    n235 = for {
      tunnel: w224 -> [w921] mode=indexing
      tunnel: w212 -> [w925]
      shift-right: [w922] -> w213
      shift-left: w221 -> [w923]
      # "ChipID"
      n236 = Index Array "Index Array"(array=w921) -> (element #1=w918:u16, element #2=w920:u16, element #3=w919:u16)  [unwired: 3 in]
      n237 = Equal?(x=w925, y=w918) -> (x = y?=w924:bool)
      n238 = case shown="True" w924 {
        tunnel: w923 -> [w926 w931]
        tunnel: [w926 w930] -> w922
        tunnel: w920 -> [_ w929]
        tunnel: w919 -> [_ w927]
        frame False {
          # "This event is not from selected ChipID: skip"
        }
        frame True {
          # "array 100px"
          # "Pixel number"
          # "Trigger Data"
          # "Event to record: classify trigger data according to the pixel"
          n239 = To Long Integer(number=w927) -> (32bit integer=w928:i32)
          n240 = in-place {
            in-place-border: w929 -> [w932]
            n241 = in-place-array #1(w931, w928) -> (w934:cluster{"1px Trigger Data":u16[]})
            n242 = in-place {
              in-place-border: w932 -> [w936]
              n243 = in-place-cluster #2(w934) -> ("1px Trigger Data"=w937:u16[])
              n244 = Build Array (concatenate) "Build Array"(w937, w936) -> (w935:u16[])
              n245 = in-place-cluster #2("1px Trigger Data"=w935) -> (w933:cluster{"1px Trigger Data":u16[]})
            }
            n246 = in-place-array #1(w933) -> (w930:cluster{"1px Trigger Data":u16[]}[])  [unwired: 1 out]
          }
        }
      }
    }
    "100px Trigger Data" <- w213
    n247 = for {
      tunnel: w213 -> [w611] mode=indexing
      shift-right: [w604] -> w219
      shift-left: u32 0 -> [w603]
      tunnel: w202 -> [w596] mode=indexing
      i -> [w610]
      w599 = u32 13290186  # color px bo
      w598 = u32 16762052  # color px dolent
      w607 = u16[] [7, 6, 5, 6, 8, 6, 10, 8, 10, 10]  # Test values
      w606 = FALSE  # T = test values
      # "BackGround color histogrames"
      # "Total number of events"
      # "number of events"
      # "Valors d'un pixel histogram"
      # "For each pixel: show trigger data histogram"
      n248 = Unbundle By Name(w611) -> ("1px Trigger Data"=w605:u16[])
      n249 = Select(t=w607, s=w606, f=w605) -> (s? t:f=w608:u16[])
      n250 = Array Size(array=w605) -> (size(s)=w602:i32)
      n251 = Array Max & Min(array=w608) -> (max value=w614:u16, min value=w613:u16)  [unwired: 2 out]
      n252 = To Unsigned Long Integer(number=w602) -> (unsigned 32bit integer=w601:u32)
      n253 = Subtract(x=w614, y=w613) -> (x-y=w612:u16)
      n254 = Increment(x=w612) -> (x+1=w616:u16)
      n255 = Add(x=w601, y=w603) -> (x+y=w604:u32)
      n256 = To Long Integer(number=w616) -> (32bit integer=w617:i32)
      n257 = To Double Precision Float(number=w608) -> (double precision float=w615:dbl[])
      n258 = call <vilib>:"Histogram.vi"("intervals"=w617, "X"=w615) -> ("Histogram Graph"=w609:T1)  [unwired: 6 in, 3 out]
      n259 = Select(t=w598, s=w596, f=w599) -> (s? t:f=w597:u32)
      n260 = Number To Decimal String(number=w601) -> (decimal integer string=w600:string)  [unwired: 1 in]
      n261 = case "100x indicadors histograma" shown="99" w610 {
        tunnel: w609 -> [_ w620 w623 w626 w629 w632 w635 w638 w641 w644 w647 w650 w653 w656 w659 w662 w665 w668 w671 w674 w677 w680 w683 w686 w689 w692 w695 w698 w701 w704 w707 w710 w713 w716 w719 w722 w725 w728 w731 w734 w737 w740 w743 w746 w749 w752 w755 w758 w761 w764 w767 w770 w773 w776 w779 w782 w785 w788 w791 w794 w797 w800 w803 w806 w809 w812 w815 w818 w821 w824 w827 w830 w833 w836 w839 w842 w845 w848 w851 w854 w857 w860 w863 w866 w869 w872 w875 w878 w881 w884 w887 w890 w893 w896 w899 w902 w905 w908 w911 w914 w917]
        tunnel: w600 -> [_ w619 w622 w625 w628 w631 w634 w637 w640 w643 w646 w649 w652 w655 w658 w661 w664 w667 w670 w673 w676 w679 w682 w685 w688 w691 w694 w697 w700 w703 w706 w709 w712 w715 w718 w721 w724 w727 w730 w733 w736 w739 w742 w745 w748 w751 w754 w757 w760 w763 w766 w769 w772 w775 w778 w781 w784 w787 w790 w793 w796 w799 w802 w805 w808 w811 w814 w817 w820 w823 w826 w829 w832 w835 w838 w841 w844 w847 w850 w853 w856 w859 w862 w865 w868 w871 w874 w877 w880 w883 w886 w889 w892 w895 w898 w901 w904 w907 w910 w913 w916]
        tunnel: w597 -> [_ w618 w621 w624 w627 w630 w633 w636 w639 w642 w645 w648 w651 w654 w657 w660 w663 w666 w669 w672 w675 w678 w681 w684 w687 w690 w693 w696 w699 w702 w705 w708 w711 w714 w717 w720 w723 w726 w729 w732 w735 w738 w741 w744 w747 w750 w753 w756 w759 w762 w765 w768 w771 w774 w777 w780 w783 w786 w789 w792 w795 w798 w801 w804 w807 w810 w813 w816 w819 w822 w825 w828 w831 w834 w837 w840 w843 w846 w849 w852 w855 w858 w861 w864 w867 w870 w873 w876 w879 w882 w885 w888 w891 w894 w897 w900 w903 w906 w909 w912 w915]
        frame Default {
        }
        frame 0 {
          n262 = property on="Trigger histogram 00" class="XYGraph (strict)"("TipStrip"=w619, "BG Color"=w618) -> ()  [unwired: 2 in, 2 out]
          "Trigger histogram 00" <- w620
        }
        frame 1 {
          n263 = property on="Trigger histogram 01" class="XYGraph (strict)"("TipStrip"=w622, "BG Color"=w621) -> ()  [unwired: 2 in, 2 out]
          "Trigger histogram 01" <- w623
        }
        frame 2 {
          n264 = property on="Trigger histogram 02" class="XYGraph (strict)"("TipStrip"=w625, "BG Color"=w624) -> ()  [unwired: 2 in, 2 out]
          "Trigger histogram 02" <- w626
        }
        frame 3 {
          n265 = property on="Trigger histogram 03" class="XYGraph (strict)"("TipStrip"=w628, "BG Color"=w627) -> ()  [unwired: 2 in, 2 out]
          "Trigger histogram 03" <- w629
        }
        frame 4 {
          n266 = property on="Trigger histogram 04" class="XYGraph (strict)"("TipStrip"=w631, "BG Color"=w630) -> ()  [unwired: 2 in, 2 out]
          "Trigger histogram 04" <- w632
        }
        frame 5 {
          n267 = property on="Trigger histogram 05" class="XYGraph (strict)"("TipStrip"=w634, "BG Color"=w633) -> ()  [unwired: 2 in, 2 out]
          "Trigger histogram 05" <- w635
        }
        frame 6 {
          n268 = property on="Trigger histogram 06" class="XYGraph (strict)"("TipStrip"=w637, "BG Color"=w636) -> ()  [unwired: 2 in, 2 out]
          "Trigger histogram 06" <- w638
        }
        frame 7 {
          n269 = property on="Trigger histogram 07" class="XYGraph (strict)"("TipStrip"=w640, "BG Color"=w639) -> ()  [unwired: 2 in, 2 out]
          "Trigger histogram 07" <- w641
        }
        frame 8 {
          n270 = property on="Trigger histogram 08" class="XYGraph (strict)"("TipStrip"=w643, "BG Color"=w642) -> ()  [unwired: 2 in, 2 out]
          "Trigger histogram 08" <- w644
        }
        frame 9 {
          n271 = property on="Trigger histogram 09" class="XYGraph (strict)"("TipStrip"=w646, "BG Color"=w645) -> ()  [unwired: 2 in, 2 out]
          "Trigger histogram 09" <- w647
        }
        frame 10 {
          n272 = property on="Trigger histogram 10" class="XYGraph (strict)"("TipStrip"=w649, "BG Color"=w648) -> ()  [unwired: 2 in, 2 out]
          "Trigger histogram 10" <- w650
        }
        frame 11 {
          n273 = property on="Trigger histogram 11" class="XYGraph (strict)"("TipStrip"=w652, "BG Color"=w651) -> ()  [unwired: 2 in, 2 out]
          "Trigger histogram 11" <- w653
        }
        frame 12 {
          n274 = property on="Trigger histogram 12" class="XYGraph (strict)"("TipStrip"=w655, "BG Color"=w654) -> ()  [unwired: 2 in, 2 out]
          "Trigger histogram 12" <- w656
        }
        frame 13 {
          n275 = property on="Trigger histogram 13" class="XYGraph (strict)"("TipStrip"=w658, "BG Color"=w657) -> ()  [unwired: 2 in, 2 out]
          "Trigger histogram 13" <- w659
        }
        frame 14 {
          n276 = property on="Trigger histogram 14" class="XYGraph (strict)"("TipStrip"=w661, "BG Color"=w660) -> ()  [unwired: 2 in, 2 out]
          "Trigger histogram 14" <- w662
        }
        frame 15 {
          n277 = property on="Trigger histogram 15" class="XYGraph (strict)"("TipStrip"=w664, "BG Color"=w663) -> ()  [unwired: 2 in, 2 out]
          "Trigger histogram 15" <- w665
        }
        frame 16 {
          n278 = property on="Trigger histogram 16" class="XYGraph (strict)"("TipStrip"=w667, "BG Color"=w666) -> ()  [unwired: 2 in, 2 out]
          "Trigger histogram 16" <- w668
        }
        frame 17 {
          n279 = property on="Trigger histogram 17" class="XYGraph (strict)"("TipStrip"=w670, "BG Color"=w669) -> ()  [unwired: 2 in, 2 out]
          "Trigger histogram 17" <- w671
        }
        frame 18 {
          n280 = property on="Trigger histogram 18" class="XYGraph (strict)"("TipStrip"=w673, "BG Color"=w672) -> ()  [unwired: 2 in, 2 out]
          "Trigger histogram 18" <- w674
        }
        frame 19 {
          n281 = property on="Trigger histogram 19" class="XYGraph (strict)"("TipStrip"=w676, "BG Color"=w675) -> ()  [unwired: 2 in, 2 out]
          "Trigger histogram 19" <- w677
        }
        frame 20 {
          n282 = property on="Trigger histogram 20" class="XYGraph (strict)"("TipStrip"=w679, "BG Color"=w678) -> ()  [unwired: 2 in, 2 out]
          "Trigger histogram 20" <- w680
        }
        frame 21 {
          n283 = property on="Trigger histogram 21" class="XYGraph (strict)"("TipStrip"=w682, "BG Color"=w681) -> ()  [unwired: 2 in, 2 out]
          "Trigger histogram 21" <- w683
        }
        frame 22 {
          n284 = property on="Trigger histogram 22" class="XYGraph (strict)"("TipStrip"=w685, "BG Color"=w684) -> ()  [unwired: 2 in, 2 out]
          "Trigger histogram 22" <- w686
        }
        frame 23 {
          n285 = property on="Trigger histogram 23" class="XYGraph (strict)"("TipStrip"=w688, "BG Color"=w687) -> ()  [unwired: 2 in, 2 out]
          "Trigger histogram 23" <- w689
        }
        frame 24 {
          n286 = property on="Trigger histogram 24" class="XYGraph (strict)"("TipStrip"=w691, "BG Color"=w690) -> ()  [unwired: 2 in, 2 out]
          "Trigger histogram 24" <- w692
        }
        frame 25 {
          n287 = property on="Trigger histogram 25" class="XYGraph (strict)"("TipStrip"=w694, "BG Color"=w693) -> ()  [unwired: 2 in, 2 out]
          "Trigger histogram 25" <- w695
        }
        frame 26 {
          n288 = property on="Trigger histogram 26" class="XYGraph (strict)"("TipStrip"=w697, "BG Color"=w696) -> ()  [unwired: 2 in, 2 out]
          "Trigger histogram 26" <- w698
        }
        frame 27 {
          n289 = property on="Trigger histogram 27" class="XYGraph (strict)"("TipStrip"=w700, "BG Color"=w699) -> ()  [unwired: 2 in, 2 out]
          "Trigger histogram 27" <- w701
        }
        frame 28 {
          n290 = property on="Trigger histogram 28" class="XYGraph (strict)"("TipStrip"=w703, "BG Color"=w702) -> ()  [unwired: 2 in, 2 out]
          "Trigger histogram 28" <- w704
        }
        frame 29 {
          n291 = property on="Trigger histogram 29" class="XYGraph (strict)"("TipStrip"=w706, "BG Color"=w705) -> ()  [unwired: 2 in, 2 out]
          "Trigger histogram 29" <- w707
        }
        frame 30 {
          n292 = property on="Trigger histogram 30" class="XYGraph (strict)"("TipStrip"=w709, "BG Color"=w708) -> ()  [unwired: 2 in, 2 out]
          "Trigger histogram 30" <- w710
        }
        frame 31 {
          n293 = property on="Trigger histogram 31" class="XYGraph (strict)"("TipStrip"=w712, "BG Color"=w711) -> ()  [unwired: 2 in, 2 out]
          "Trigger histogram 31" <- w713
        }
        frame 32 {
          n294 = property on="Trigger histogram 32" class="XYGraph (strict)"("TipStrip"=w715, "BG Color"=w714) -> ()  [unwired: 2 in, 2 out]
          "Trigger histogram 32" <- w716
        }
        frame 33 {
          n295 = property on="Trigger histogram 33" class="XYGraph (strict)"("TipStrip"=w718, "BG Color"=w717) -> ()  [unwired: 2 in, 2 out]
          "Trigger histogram 33" <- w719
        }
        frame 34 {
          n296 = property on="Trigger histogram 34" class="XYGraph (strict)"("TipStrip"=w721, "BG Color"=w720) -> ()  [unwired: 2 in, 2 out]
          "Trigger histogram 34" <- w722
        }
        frame 35 {
          n297 = property on="Trigger histogram 35" class="XYGraph (strict)"("TipStrip"=w724, "BG Color"=w723) -> ()  [unwired: 2 in, 2 out]
          "Trigger histogram 35" <- w725
        }
        frame 36 {
          n298 = property on="Trigger histogram 36" class="XYGraph (strict)"("TipStrip"=w727, "BG Color"=w726) -> ()  [unwired: 2 in, 2 out]
          "Trigger histogram 36" <- w728
        }
        frame 37 {
          n299 = property on="Trigger histogram 37" class="XYGraph (strict)"("TipStrip"=w730, "BG Color"=w729) -> ()  [unwired: 2 in, 2 out]
          "Trigger histogram 37" <- w731
        }
        frame 38 {
          n300 = property on="Trigger histogram 38" class="XYGraph (strict)"("TipStrip"=w733, "BG Color"=w732) -> ()  [unwired: 2 in, 2 out]
          "Trigger histogram 38" <- w734
        }
        frame 39 {
          n301 = property on="Trigger histogram 39" class="XYGraph (strict)"("TipStrip"=w736, "BG Color"=w735) -> ()  [unwired: 2 in, 2 out]
          "Trigger histogram 39" <- w737
        }
        frame 40 {
          n302 = property on="Trigger histogram 40" class="XYGraph (strict)"("TipStrip"=w739, "BG Color"=w738) -> ()  [unwired: 2 in, 2 out]
          "Trigger histogram 40" <- w740
        }
        frame 41 {
          n303 = property on="Trigger histogram 41" class="XYGraph (strict)"("TipStrip"=w742, "BG Color"=w741) -> ()  [unwired: 2 in, 2 out]
          "Trigger histogram 41" <- w743
        }
        frame 42 {
          n304 = property on="Trigger histogram 42" class="XYGraph (strict)"("TipStrip"=w745, "BG Color"=w744) -> ()  [unwired: 2 in, 2 out]
          "Trigger histogram 42" <- w746
        }
        frame 43 {
          n305 = property on="Trigger histogram 43" class="XYGraph (strict)"("TipStrip"=w748, "BG Color"=w747) -> ()  [unwired: 2 in, 2 out]
          "Trigger histogram 43" <- w749
        }
        frame 44 {
          n306 = property on="Trigger histogram 44" class="XYGraph (strict)"("TipStrip"=w751, "BG Color"=w750) -> ()  [unwired: 2 in, 2 out]
          "Trigger histogram 44" <- w752
        }
        frame 45 {
          n307 = property on="Trigger histogram 45" class="XYGraph (strict)"("TipStrip"=w754, "BG Color"=w753) -> ()  [unwired: 2 in, 2 out]
          "Trigger histogram 45" <- w755
        }
        frame 46 {
          n308 = property on="Trigger histogram 46" class="XYGraph (strict)"("TipStrip"=w757, "BG Color"=w756) -> ()  [unwired: 2 in, 2 out]
          "Trigger histogram 46" <- w758
        }
        frame 47 {
          n309 = property on="Trigger histogram 47" class="XYGraph (strict)"("TipStrip"=w760, "BG Color"=w759) -> ()  [unwired: 2 in, 2 out]
          "Trigger histogram 47" <- w761
        }
        frame 48 {
          n310 = property on="Trigger histogram 48" class="XYGraph (strict)"("TipStrip"=w763, "BG Color"=w762) -> ()  [unwired: 2 in, 2 out]
          "Trigger histogram 48" <- w764
        }
        frame 49 {
          n311 = property on="Trigger histogram 49" class="XYGraph (strict)"("TipStrip"=w766, "BG Color"=w765) -> ()  [unwired: 2 in, 2 out]
          "Trigger histogram 49" <- w767
        }
        frame 50 {
          n312 = property on="Trigger histogram 50" class="XYGraph (strict)"("TipStrip"=w769, "BG Color"=w768) -> ()  [unwired: 2 in, 2 out]
          "Trigger histogram 50" <- w770
        }
        frame 51 {
          n313 = property on="Trigger histogram 51" class="XYGraph (strict)"("TipStrip"=w772, "BG Color"=w771) -> ()  [unwired: 2 in, 2 out]
          "Trigger histogram 51" <- w773
        }
        frame 52 {
          n314 = property on="Trigger histogram 52" class="XYGraph (strict)"("TipStrip"=w775, "BG Color"=w774) -> ()  [unwired: 2 in, 2 out]
          "Trigger histogram 52" <- w776
        }
        frame 53 {
          n315 = property on="Trigger histogram 53" class="XYGraph (strict)"("TipStrip"=w778, "BG Color"=w777) -> ()  [unwired: 2 in, 2 out]
          "Trigger histogram 53" <- w779
        }
        frame 54 {
          n316 = property on="Trigger histogram 54" class="XYGraph (strict)"("TipStrip"=w781, "BG Color"=w780) -> ()  [unwired: 2 in, 2 out]
          "Trigger histogram 54" <- w782
        }
        frame 55 {
          n317 = property on="Trigger histogram 55" class="XYGraph (strict)"("TipStrip"=w784, "BG Color"=w783) -> ()  [unwired: 2 in, 2 out]
          "Trigger histogram 55" <- w785
        }
        frame 56 {
          n318 = property on="Trigger histogram 56" class="XYGraph (strict)"("TipStrip"=w787, "BG Color"=w786) -> ()  [unwired: 2 in, 2 out]
          "Trigger histogram 56" <- w788
        }
        frame 57 {
          n319 = property on="Trigger histogram 57" class="XYGraph (strict)"("TipStrip"=w790, "BG Color"=w789) -> ()  [unwired: 2 in, 2 out]
          "Trigger histogram 57" <- w791
        }
        frame 58 {
          n320 = property on="Trigger histogram 58" class="XYGraph (strict)"("TipStrip"=w793, "BG Color"=w792) -> ()  [unwired: 2 in, 2 out]
          "Trigger histogram 58" <- w794
        }
        frame 59 {
          n321 = property on="Trigger histogram 59" class="XYGraph (strict)"("TipStrip"=w796, "BG Color"=w795) -> ()  [unwired: 2 in, 2 out]
          "Trigger histogram 59" <- w797
        }
        frame 60 {
          n322 = property on="Trigger histogram 60" class="XYGraph (strict)"("TipStrip"=w799, "BG Color"=w798) -> ()  [unwired: 2 in, 2 out]
          "Trigger histogram 60" <- w800
        }
        frame 61 {
          n323 = property on="Trigger histogram 61" class="XYGraph (strict)"("TipStrip"=w802, "BG Color"=w801) -> ()  [unwired: 2 in, 2 out]
          "Trigger histogram 61" <- w803
        }
        frame 62 {
          n324 = property on="Trigger histogram 62" class="XYGraph (strict)"("TipStrip"=w805, "BG Color"=w804) -> ()  [unwired: 2 in, 2 out]
          "Trigger histogram 62" <- w806
        }
        frame 63 {
          n325 = property on="Trigger histogram 63" class="XYGraph (strict)"("TipStrip"=w808, "BG Color"=w807) -> ()  [unwired: 2 in, 2 out]
          "Trigger histogram 63" <- w809
        }
        frame 64 {
          n326 = property on="Trigger histogram 64" class="XYGraph (strict)"("TipStrip"=w811, "BG Color"=w810) -> ()  [unwired: 2 in, 2 out]
          "Trigger histogram 64" <- w812
        }
        frame 65 {
          n327 = property on="Trigger histogram 65" class="XYGraph (strict)"("TipStrip"=w814, "BG Color"=w813) -> ()  [unwired: 2 in, 2 out]
          "Trigger histogram 65" <- w815
        }
        frame 66 {
          n328 = property on="Trigger histogram 66" class="XYGraph (strict)"("TipStrip"=w817, "BG Color"=w816) -> ()  [unwired: 2 in, 2 out]
          "Trigger histogram 66" <- w818
        }
        frame 67 {
          n329 = property on="Trigger histogram 67" class="XYGraph (strict)"("TipStrip"=w820, "BG Color"=w819) -> ()  [unwired: 2 in, 2 out]
          "Trigger histogram 67" <- w821
        }
        frame 68 {
          n330 = property on="Trigger histogram 68" class="XYGraph (strict)"("TipStrip"=w823, "BG Color"=w822) -> ()  [unwired: 2 in, 2 out]
          "Trigger histogram 68" <- w824
        }
        frame 69 {
          n331 = property on="Trigger histogram 69" class="XYGraph (strict)"("TipStrip"=w826, "BG Color"=w825) -> ()  [unwired: 2 in, 2 out]
          "Trigger histogram 69" <- w827
        }
        frame 70 {
          n332 = property on="Trigger histogram 70" class="XYGraph (strict)"("TipStrip"=w829, "BG Color"=w828) -> ()  [unwired: 2 in, 2 out]
          "Trigger histogram 70" <- w830
        }
        frame 71 {
          n333 = property on="Trigger histogram 71" class="XYGraph (strict)"("TipStrip"=w832, "BG Color"=w831) -> ()  [unwired: 2 in, 2 out]
          "Trigger histogram 71" <- w833
        }
        frame 72 {
          n334 = property on="Trigger histogram 72" class="XYGraph (strict)"("TipStrip"=w835, "BG Color"=w834) -> ()  [unwired: 2 in, 2 out]
          "Trigger histogram 72" <- w836
        }
        frame 73 {
          n335 = property on="Trigger histogram 73" class="XYGraph (strict)"("TipStrip"=w838, "BG Color"=w837) -> ()  [unwired: 2 in, 2 out]
          "Trigger histogram 73" <- w839
        }
        frame 74 {
          n336 = property on="Trigger histogram 74" class="XYGraph (strict)"("TipStrip"=w841, "BG Color"=w840) -> ()  [unwired: 2 in, 2 out]
          "Trigger histogram 74" <- w842
        }
        frame 75 {
          n337 = property on="Trigger histogram 75" class="XYGraph (strict)"("TipStrip"=w844, "BG Color"=w843) -> ()  [unwired: 2 in, 2 out]
          "Trigger histogram 75" <- w845
        }
        frame 76 {
          n338 = property on="Trigger histogram 76" class="XYGraph (strict)"("TipStrip"=w847, "BG Color"=w846) -> ()  [unwired: 2 in, 2 out]
          "Trigger histogram 76" <- w848
        }
        frame 77 {
          n339 = property on="Trigger histogram 77" class="XYGraph (strict)"("TipStrip"=w850, "BG Color"=w849) -> ()  [unwired: 2 in, 2 out]
          "Trigger histogram 77" <- w851
        }
        frame 78 {
          n340 = property on="Trigger histogram 78" class="XYGraph (strict)"("TipStrip"=w853, "BG Color"=w852) -> ()  [unwired: 2 in, 2 out]
          "Trigger histogram 78" <- w854
        }
        frame 79 {
          n341 = property on="Trigger histogram 79" class="XYGraph (strict)"("TipStrip"=w856, "BG Color"=w855) -> ()  [unwired: 2 in, 2 out]
          "Trigger histogram 79" <- w857
        }
        frame 80 {
          n342 = property on="Trigger histogram 80" class="XYGraph (strict)"("TipStrip"=w859, "BG Color"=w858) -> ()  [unwired: 2 in, 2 out]
          "Trigger histogram 80" <- w860
        }
        frame 81 {
          n343 = property on="Trigger histogram 81" class="XYGraph (strict)"("TipStrip"=w862, "BG Color"=w861) -> ()  [unwired: 2 in, 2 out]
          "Trigger histogram 81" <- w863
        }
        frame 82 {
          n344 = property on="Trigger histogram 82" class="XYGraph (strict)"("TipStrip"=w865, "BG Color"=w864) -> ()  [unwired: 2 in, 2 out]
          "Trigger histogram 82" <- w866
        }
        frame 83 {
          n345 = property on="Trigger histogram 83" class="XYGraph (strict)"("TipStrip"=w868, "BG Color"=w867) -> ()  [unwired: 2 in, 2 out]
          "Trigger histogram 83" <- w869
        }
        frame 84 {
          n346 = property on="Trigger histogram 84" class="XYGraph (strict)"("TipStrip"=w871, "BG Color"=w870) -> ()  [unwired: 2 in, 2 out]
          "Trigger histogram 84" <- w872
        }
        frame 85 {
          n347 = property on="Trigger histogram 85" class="XYGraph (strict)"("TipStrip"=w874, "BG Color"=w873) -> ()  [unwired: 2 in, 2 out]
          "Trigger histogram 85" <- w875
        }
        frame 86 {
          n348 = property on="Trigger histogram 86" class="XYGraph (strict)"("TipStrip"=w877, "BG Color"=w876) -> ()  [unwired: 2 in, 2 out]
          "Trigger histogram 86" <- w878
        }
        frame 87 {
          n349 = property on="Trigger histogram 87" class="XYGraph (strict)"("TipStrip"=w880, "BG Color"=w879) -> ()  [unwired: 2 in, 2 out]
          "Trigger histogram 87" <- w881
        }
        frame 88 {
          n350 = property on="Trigger histogram 88" class="XYGraph (strict)"("TipStrip"=w883, "BG Color"=w882) -> ()  [unwired: 2 in, 2 out]
          "Trigger histogram 88" <- w884
        }
        frame 89 {
          n351 = property on="Trigger histogram 89" class="XYGraph (strict)"("TipStrip"=w886, "BG Color"=w885) -> ()  [unwired: 2 in, 2 out]
          "Trigger histogram 89" <- w887
        }
        frame 90 {
          n352 = property on="Trigger histogram 90" class="XYGraph (strict)"("TipStrip"=w889, "BG Color"=w888) -> ()  [unwired: 2 in, 2 out]
          "Trigger histogram 90" <- w890
        }
        frame 91 {
          n353 = property on="Trigger histogram 91" class="XYGraph (strict)"("TipStrip"=w892, "BG Color"=w891) -> ()  [unwired: 2 in, 2 out]
          "Trigger histogram 91" <- w893
        }
        frame 92 {
          n354 = property on="Trigger histogram 92" class="XYGraph (strict)"("TipStrip"=w895, "BG Color"=w894) -> ()  [unwired: 2 in, 2 out]
          "Trigger histogram 92" <- w896
        }
        frame 93 {
          n355 = property on="Trigger histogram 93" class="XYGraph (strict)"("TipStrip"=w898, "BG Color"=w897) -> ()  [unwired: 2 in, 2 out]
          "Trigger histogram 93" <- w899
        }
        frame 94 {
          n356 = property on="Trigger histogram 94" class="XYGraph (strict)"("TipStrip"=w901, "BG Color"=w900) -> ()  [unwired: 2 in, 2 out]
          "Trigger histogram 94" <- w902
        }
        frame 95 {
          n357 = property on="Trigger histogram 95" class="XYGraph (strict)"("TipStrip"=w904, "BG Color"=w903) -> ()  [unwired: 2 in, 2 out]
          "Trigger histogram 95" <- w905
        }
        frame 96 {
          n358 = property on="Trigger histogram 96" class="XYGraph (strict)"("TipStrip"=w907, "BG Color"=w906) -> ()  [unwired: 2 in, 2 out]
          "Trigger histogram 96" <- w908
        }
        frame 97 {
          n359 = property on="Trigger histogram 97" class="XYGraph (strict)"("TipStrip"=w910, "BG Color"=w909) -> ()  [unwired: 2 in, 2 out]
          "Trigger histogram 97" <- w911
        }
        frame 98 {
          n360 = property on="Trigger histogram 98" class="XYGraph (strict)"("TipStrip"=w913, "BG Color"=w912) -> ()  [unwired: 2 in, 2 out]
          "Trigger histogram 98" <- w914
        }
        frame 99 {
          n361 = property on="Trigger histogram 99" class="XYGraph (strict)"("TipStrip"=w916, "BG Color"=w915) -> ()  [unwired: 2 in, 2 out]
          "Trigger histogram 99" <- w917
        }
      }
    }
    n362 = flat-sequence {
      tunnel: w219 -> [w266]
      tunnel: [w267] -> w218
      frame #0 {
        "Total number of events" <- w266
      }
      frame #1 {
        # "User interactions: buttons"
        n363 = while {
          tunnel: [w269] -> w267
          stop <- w268 stop-if-true
          n364 = event shown="[3] \"Y scale\", \"X scale min.\", \"X scale max.\": Value Change" {
            selector: _ -> [_ _ _ _ _]
            dyn-events: _ -> [_ _ _ _ _]
            timeout: _ -> [_ _ _ _ _]
            tunnel: [_ w270 w272 w277 w582] -> w269
            tunnel: [_ w270 TRUE ("Close viewer") w277 w582] -> w268
            event Timeout {
              n365 = event-data() -> ()  [unwired: 1 in, 2 out]
            }
            event "Close button": Mouse Down {
              w270 = TRUE  # Close viewer
              n366 = event-data() -> ()  [unwired: 1 in, 7 out]
            }
            event "Choose Chip button": Mouse Down {
              w272 = FALSE  # Another iteration: choose ChipID
              n367 = event-data() -> ()  [unwired: 1 in, 7 out]
            }
            event "Y scale", "X scale min.", "X scale max.": Value Change {
              w277 = FALSE ("Close viewer")
              n368 = event-data() -> ()  [unwired: 1 in, 5 out]
              n369 = for {
                N: 100 -> [_]
                tunnel: "Y scale" -> [w280]
                tunnel: "X scale min." -> [w279]
                tunnel: "X scale max." -> [w278]
                i -> [w281]
                # "Fix Scales"
                n370 = case shown="0" w281 {
                  tunnel: w280 -> [_ w284 w287 w290 w293 w296 w299 w302 w305 w308 w311 w314 w317 w320 w323 w326 w329 w332 w335 w338 w341 w344 w347 w350 w353 w356 w359 w362 w365 w368 w371 w374 w377 w380 w383 w386 w389 w392 w395 w398 w401 w404 w407 w410 w413 w416 w419 w422 w425 w428 w431 w434 w437 w440 w443 w446 w449 w452 w455 w458 w461 w464 w467 w470 w473 w476 w479 w482 w485 w488 w491 w494 w497 w500 w503 w506 w509 w512 w515 w518 w521 w524 w527 w530 w533 w536 w539 w542 w545 w548 w551 w554 w557 w560 w563 w566 w569 w572 w575 w578 w581]
                  tunnel: w279 -> [_ w283 w286 w289 w292 w295 w298 w301 w304 w307 w310 w313 w316 w319 w322 w325 w328 w331 w334 w337 w340 w343 w346 w349 w352 w355 w358 w361 w364 w367 w370 w373 w376 w379 w382 w385 w388 w391 w394 w397 w400 w403 w406 w409 w412 w415 w418 w421 w424 w427 w430 w433 w436 w439 w442 w445 w448 w451 w454 w457 w460 w463 w466 w469 w472 w475 w478 w481 w484 w487 w490 w493 w496 w499 w502 w505 w508 w511 w514 w517 w520 w523 w526 w529 w532 w535 w538 w541 w544 w547 w550 w553 w556 w559 w562 w565 w568 w571 w574 w577 w580]
                  tunnel: w278 -> [_ w282 w285 w288 w291 w294 w297 w300 w303 w306 w309 w312 w315 w318 w321 w324 w327 w330 w333 w336 w339 w342 w345 w348 w351 w354 w357 w360 w363 w366 w369 w372 w375 w378 w381 w384 w387 w390 w393 w396 w399 w402 w405 w408 w411 w414 w417 w420 w423 w426 w429 w432 w435 w438 w441 w444 w447 w450 w453 w456 w459 w462 w465 w468 w471 w474 w477 w480 w483 w486 w489 w492 w495 w498 w501 w504 w507 w510 w513 w516 w519 w522 w525 w528 w531 w534 w537 w540 w543 w546 w549 w552 w555 w558 w561 w564 w567 w570 w573 w576 w579]
                  frame Default {
                  }
                  frame 0 {
                    n371 = property on="Trigger histogram 00" class="XYGraph (strict)"("YScale.Maximum"=w284, "XScale.Minimum"=w283, "XScale.Maximum"=w282) -> ()  [unwired: 2 in, 2 out]
                  }
                  frame 1 {
                    n372 = property on="Trigger histogram 01" class="XYGraph (strict)"("YScale.Maximum"=w287, "XScale.Minimum"=w286, "XScale.Maximum"=w285) -> ()  [unwired: 2 in, 2 out]
                  }
                  frame 2 {
                    n373 = property on="Trigger histogram 02" class="XYGraph (strict)"("YScale.Maximum"=w290, "XScale.Minimum"=w289, "XScale.Maximum"=w288) -> ()  [unwired: 2 in, 2 out]
                  }
                  frame 3 {
                    n374 = property on="Trigger histogram 03" class="XYGraph (strict)"("YScale.Maximum"=w293, "XScale.Minimum"=w292, "XScale.Maximum"=w291) -> ()  [unwired: 2 in, 2 out]
                  }
                  frame 4 {
                    n375 = property on="Trigger histogram 04" class="XYGraph (strict)"("YScale.Maximum"=w296, "XScale.Minimum"=w295, "XScale.Maximum"=w294) -> ()  [unwired: 2 in, 2 out]
                  }
                  frame 5 {
                    n376 = property on="Trigger histogram 05" class="XYGraph (strict)"("YScale.Maximum"=w299, "XScale.Minimum"=w298, "XScale.Maximum"=w297) -> ()  [unwired: 2 in, 2 out]
                  }
                  frame 6 {
                    n377 = property on="Trigger histogram 06" class="XYGraph (strict)"("YScale.Maximum"=w302, "XScale.Minimum"=w301, "XScale.Maximum"=w300) -> ()  [unwired: 2 in, 2 out]
                  }
                  frame 7 {
                    n378 = property on="Trigger histogram 07" class="XYGraph (strict)"("YScale.Maximum"=w305, "XScale.Minimum"=w304, "XScale.Maximum"=w303) -> ()  [unwired: 2 in, 2 out]
                  }
                  frame 8 {
                    n379 = property on="Trigger histogram 08" class="XYGraph (strict)"("YScale.Maximum"=w308, "XScale.Minimum"=w307, "XScale.Maximum"=w306) -> ()  [unwired: 2 in, 2 out]
                  }
                  frame 9 {
                    n380 = property on="Trigger histogram 09" class="XYGraph (strict)"("YScale.Maximum"=w311, "XScale.Minimum"=w310, "XScale.Maximum"=w309) -> ()  [unwired: 2 in, 2 out]
                  }
                  frame 10 {
                    n381 = property on="Trigger histogram 10" class="XYGraph (strict)"("YScale.Maximum"=w314, "XScale.Minimum"=w313, "XScale.Maximum"=w312) -> ()  [unwired: 2 in, 2 out]
                  }
                  frame 11 {
                    n382 = property on="Trigger histogram 11" class="XYGraph (strict)"("YScale.Maximum"=w317, "XScale.Minimum"=w316, "XScale.Maximum"=w315) -> ()  [unwired: 2 in, 2 out]
                  }
                  frame 12 {
                    n383 = property on="Trigger histogram 12" class="XYGraph (strict)"("YScale.Maximum"=w320, "XScale.Minimum"=w319, "XScale.Maximum"=w318) -> ()  [unwired: 2 in, 2 out]
                  }
                  frame 13 {
                    n384 = property on="Trigger histogram 13" class="XYGraph (strict)"("YScale.Maximum"=w323, "XScale.Minimum"=w322, "XScale.Maximum"=w321) -> ()  [unwired: 2 in, 2 out]
                  }
                  frame 14 {
                    n385 = property on="Trigger histogram 14" class="XYGraph (strict)"("YScale.Maximum"=w326, "XScale.Minimum"=w325, "XScale.Maximum"=w324) -> ()  [unwired: 2 in, 2 out]
                  }
                  frame 15 {
                    n386 = property on="Trigger histogram 15" class="XYGraph (strict)"("YScale.Maximum"=w329, "XScale.Minimum"=w328, "XScale.Maximum"=w327) -> ()  [unwired: 2 in, 2 out]
                  }
                  frame 16 {
                    n387 = property on="Trigger histogram 16" class="XYGraph (strict)"("YScale.Maximum"=w332, "XScale.Minimum"=w331, "XScale.Maximum"=w330) -> ()  [unwired: 2 in, 2 out]
                  }
                  frame 17 {
                    n388 = property on="Trigger histogram 17" class="XYGraph (strict)"("YScale.Maximum"=w335, "XScale.Minimum"=w334, "XScale.Maximum"=w333) -> ()  [unwired: 2 in, 2 out]
                  }
                  frame 18 {
                    n389 = property on="Trigger histogram 18" class="XYGraph (strict)"("YScale.Maximum"=w338, "XScale.Minimum"=w337, "XScale.Maximum"=w336) -> ()  [unwired: 2 in, 2 out]
                  }
                  frame 19 {
                    n390 = property on="Trigger histogram 19" class="XYGraph (strict)"("YScale.Maximum"=w341, "XScale.Minimum"=w340, "XScale.Maximum"=w339) -> ()  [unwired: 2 in, 2 out]
                  }
                  frame 20 {
                    n391 = property on="Trigger histogram 20" class="XYGraph (strict)"("YScale.Maximum"=w344, "XScale.Minimum"=w343, "XScale.Maximum"=w342) -> ()  [unwired: 2 in, 2 out]
                  }
                  frame 21 {
                    n392 = property on="Trigger histogram 21" class="XYGraph (strict)"("YScale.Maximum"=w347, "XScale.Minimum"=w346, "XScale.Maximum"=w345) -> ()  [unwired: 2 in, 2 out]
                  }
                  frame 22 {
                    n393 = property on="Trigger histogram 22" class="XYGraph (strict)"("YScale.Maximum"=w350, "XScale.Minimum"=w349, "XScale.Maximum"=w348) -> ()  [unwired: 2 in, 2 out]
                  }
                  frame 23 {
                    n394 = property on="Trigger histogram 23" class="XYGraph (strict)"("YScale.Maximum"=w353, "XScale.Minimum"=w352, "XScale.Maximum"=w351) -> ()  [unwired: 2 in, 2 out]
                  }
                  frame 24 {
                    n395 = property on="Trigger histogram 24" class="XYGraph (strict)"("YScale.Maximum"=w356, "XScale.Minimum"=w355, "XScale.Maximum"=w354) -> ()  [unwired: 2 in, 2 out]
                  }
                  frame 25 {
                    n396 = property on="Trigger histogram 25" class="XYGraph (strict)"("YScale.Maximum"=w359, "XScale.Minimum"=w358, "XScale.Maximum"=w357) -> ()  [unwired: 2 in, 2 out]
                  }
                  frame 26 {
                    n397 = property on="Trigger histogram 26" class="XYGraph (strict)"("YScale.Maximum"=w362, "XScale.Minimum"=w361, "XScale.Maximum"=w360) -> ()  [unwired: 2 in, 2 out]
                  }
                  frame 27 {
                    n398 = property on="Trigger histogram 27" class="XYGraph (strict)"("YScale.Maximum"=w365, "XScale.Minimum"=w364, "XScale.Maximum"=w363) -> ()  [unwired: 2 in, 2 out]
                  }
                  frame 28 {
                    n399 = property on="Trigger histogram 28" class="XYGraph (strict)"("YScale.Maximum"=w368, "XScale.Minimum"=w367, "XScale.Maximum"=w366) -> ()  [unwired: 2 in, 2 out]
                  }
                  frame 29 {
                    n400 = property on="Trigger histogram 29" class="XYGraph (strict)"("YScale.Maximum"=w371, "XScale.Minimum"=w370, "XScale.Maximum"=w369) -> ()  [unwired: 2 in, 2 out]
                  }
                  frame 30 {
                    n401 = property on="Trigger histogram 30" class="XYGraph (strict)"("YScale.Maximum"=w374, "XScale.Minimum"=w373, "XScale.Maximum"=w372) -> ()  [unwired: 2 in, 2 out]
                  }
                  frame 31 {
                    n402 = property on="Trigger histogram 31" class="XYGraph (strict)"("YScale.Maximum"=w377, "XScale.Minimum"=w376, "XScale.Maximum"=w375) -> ()  [unwired: 2 in, 2 out]
                  }
                  frame 32 {
                    n403 = property on="Trigger histogram 32" class="XYGraph (strict)"("YScale.Maximum"=w380, "XScale.Minimum"=w379, "XScale.Maximum"=w378) -> ()  [unwired: 2 in, 2 out]
                  }
                  frame 33 {
                    n404 = property on="Trigger histogram 33" class="XYGraph (strict)"("YScale.Maximum"=w383, "XScale.Minimum"=w382, "XScale.Maximum"=w381) -> ()  [unwired: 2 in, 2 out]
                  }
                  frame 34 {
                    n405 = property on="Trigger histogram 34" class="XYGraph (strict)"("YScale.Maximum"=w386, "XScale.Minimum"=w385, "XScale.Maximum"=w384) -> ()  [unwired: 2 in, 2 out]
                  }
                  frame 35 {
                    n406 = property on="Trigger histogram 35" class="XYGraph (strict)"("YScale.Maximum"=w389, "XScale.Minimum"=w388, "XScale.Maximum"=w387) -> ()  [unwired: 2 in, 2 out]
                  }
                  frame 36 {
                    n407 = property on="Trigger histogram 36" class="XYGraph (strict)"("YScale.Maximum"=w392, "XScale.Minimum"=w391, "XScale.Maximum"=w390) -> ()  [unwired: 2 in, 2 out]
                  }
                  frame 37 {
                    n408 = property on="Trigger histogram 37" class="XYGraph (strict)"("YScale.Maximum"=w395, "XScale.Minimum"=w394, "XScale.Maximum"=w393) -> ()  [unwired: 2 in, 2 out]
                  }
                  frame 38 {
                    n409 = property on="Trigger histogram 38" class="XYGraph (strict)"("YScale.Maximum"=w398, "XScale.Minimum"=w397, "XScale.Maximum"=w396) -> ()  [unwired: 2 in, 2 out]
                  }
                  frame 39 {
                    n410 = property on="Trigger histogram 39" class="XYGraph (strict)"("YScale.Maximum"=w401, "XScale.Minimum"=w400, "XScale.Maximum"=w399) -> ()  [unwired: 2 in, 2 out]
                  }
                  frame 40 {
                    n411 = property on="Trigger histogram 40" class="XYGraph (strict)"("YScale.Maximum"=w404, "XScale.Minimum"=w403, "XScale.Maximum"=w402) -> ()  [unwired: 2 in, 2 out]
                  }
                  frame 41 {
                    n412 = property on="Trigger histogram 41" class="XYGraph (strict)"("YScale.Maximum"=w407, "XScale.Minimum"=w406, "XScale.Maximum"=w405) -> ()  [unwired: 2 in, 2 out]
                  }
                  frame 42 {
                    n413 = property on="Trigger histogram 42" class="XYGraph (strict)"("YScale.Maximum"=w410, "XScale.Minimum"=w409, "XScale.Maximum"=w408) -> ()  [unwired: 2 in, 2 out]
                  }
                  frame 43 {
                    n414 = property on="Trigger histogram 43" class="XYGraph (strict)"("YScale.Maximum"=w413, "XScale.Minimum"=w412, "XScale.Maximum"=w411) -> ()  [unwired: 2 in, 2 out]
                  }
                  frame 44 {
                    n415 = property on="Trigger histogram 44" class="XYGraph (strict)"("YScale.Maximum"=w416, "XScale.Minimum"=w415, "XScale.Maximum"=w414) -> ()  [unwired: 2 in, 2 out]
                  }
                  frame 45 {
                    n416 = property on="Trigger histogram 45" class="XYGraph (strict)"("YScale.Maximum"=w419, "XScale.Minimum"=w418, "XScale.Maximum"=w417) -> ()  [unwired: 2 in, 2 out]
                  }
                  frame 46 {
                    n417 = property on="Trigger histogram 46" class="XYGraph (strict)"("YScale.Maximum"=w422, "XScale.Minimum"=w421, "XScale.Maximum"=w420) -> ()  [unwired: 2 in, 2 out]
                  }
                  frame 47 {
                    n418 = property on="Trigger histogram 47" class="XYGraph (strict)"("YScale.Maximum"=w425, "XScale.Minimum"=w424, "XScale.Maximum"=w423) -> ()  [unwired: 2 in, 2 out]
                  }
                  frame 48 {
                    n419 = property on="Trigger histogram 48" class="XYGraph (strict)"("YScale.Maximum"=w428, "XScale.Minimum"=w427, "XScale.Maximum"=w426) -> ()  [unwired: 2 in, 2 out]
                  }
                  frame 49 {
                    n420 = property on="Trigger histogram 49" class="XYGraph (strict)"("YScale.Maximum"=w431, "XScale.Minimum"=w430, "XScale.Maximum"=w429) -> ()  [unwired: 2 in, 2 out]
                  }
                  frame 50 {
                    n421 = property on="Trigger histogram 50" class="XYGraph (strict)"("YScale.Maximum"=w434, "XScale.Minimum"=w433, "XScale.Maximum"=w432) -> ()  [unwired: 2 in, 2 out]
                  }
                  frame 51 {
                    n422 = property on="Trigger histogram 51" class="XYGraph (strict)"("YScale.Maximum"=w437, "XScale.Minimum"=w436, "XScale.Maximum"=w435) -> ()  [unwired: 2 in, 2 out]
                  }
                  frame 52 {
                    n423 = property on="Trigger histogram 52" class="XYGraph (strict)"("YScale.Maximum"=w440, "XScale.Minimum"=w439, "XScale.Maximum"=w438) -> ()  [unwired: 2 in, 2 out]
                  }
                  frame 53 {
                    n424 = property on="Trigger histogram 53" class="XYGraph (strict)"("YScale.Maximum"=w443, "XScale.Minimum"=w442, "XScale.Maximum"=w441) -> ()  [unwired: 2 in, 2 out]
                  }
                  frame 54 {
                    n425 = property on="Trigger histogram 54" class="XYGraph (strict)"("YScale.Maximum"=w446, "XScale.Minimum"=w445, "XScale.Maximum"=w444) -> ()  [unwired: 2 in, 2 out]
                  }
                  frame 55 {
                    n426 = property on="Trigger histogram 55" class="XYGraph (strict)"("YScale.Maximum"=w449, "XScale.Minimum"=w448, "XScale.Maximum"=w447) -> ()  [unwired: 2 in, 2 out]
                  }
                  frame 56 {
                    n427 = property on="Trigger histogram 56" class="XYGraph (strict)"("YScale.Maximum"=w452, "XScale.Minimum"=w451, "XScale.Maximum"=w450) -> ()  [unwired: 2 in, 2 out]
                  }
                  frame 57 {
                    n428 = property on="Trigger histogram 57" class="XYGraph (strict)"("YScale.Maximum"=w455, "XScale.Minimum"=w454, "XScale.Maximum"=w453) -> ()  [unwired: 2 in, 2 out]
                  }
                  frame 58 {
                    n429 = property on="Trigger histogram 58" class="XYGraph (strict)"("YScale.Maximum"=w458, "XScale.Minimum"=w457, "XScale.Maximum"=w456) -> ()  [unwired: 2 in, 2 out]
                  }
                  frame 59 {
                    n430 = property on="Trigger histogram 59" class="XYGraph (strict)"("YScale.Maximum"=w461, "XScale.Minimum"=w460, "XScale.Maximum"=w459) -> ()  [unwired: 2 in, 2 out]
                  }
                  frame 60 {
                    n431 = property on="Trigger histogram 60" class="XYGraph (strict)"("YScale.Maximum"=w464, "XScale.Minimum"=w463, "XScale.Maximum"=w462) -> ()  [unwired: 2 in, 2 out]
                  }
                  frame 61 {
                    n432 = property on="Trigger histogram 61" class="XYGraph (strict)"("YScale.Maximum"=w467, "XScale.Minimum"=w466, "XScale.Maximum"=w465) -> ()  [unwired: 2 in, 2 out]
                  }
                  frame 62 {
                    n433 = property on="Trigger histogram 62" class="XYGraph (strict)"("YScale.Maximum"=w470, "XScale.Minimum"=w469, "XScale.Maximum"=w468) -> ()  [unwired: 2 in, 2 out]
                  }
                  frame 63 {
                    n434 = property on="Trigger histogram 63" class="XYGraph (strict)"("YScale.Maximum"=w473, "XScale.Minimum"=w472, "XScale.Maximum"=w471) -> ()  [unwired: 2 in, 2 out]
                  }
                  frame 64 {
                    n435 = property on="Trigger histogram 64" class="XYGraph (strict)"("YScale.Maximum"=w476, "XScale.Minimum"=w475, "XScale.Maximum"=w474) -> ()  [unwired: 2 in, 2 out]
                  }
                  frame 65 {
                    n436 = property on="Trigger histogram 65" class="XYGraph (strict)"("YScale.Maximum"=w479, "XScale.Minimum"=w478, "XScale.Maximum"=w477) -> ()  [unwired: 2 in, 2 out]
                  }
                  frame 66 {
                    n437 = property on="Trigger histogram 66" class="XYGraph (strict)"("YScale.Maximum"=w482, "XScale.Minimum"=w481, "XScale.Maximum"=w480) -> ()  [unwired: 2 in, 2 out]
                  }
                  frame 67 {
                    n438 = property on="Trigger histogram 67" class="XYGraph (strict)"("YScale.Maximum"=w485, "XScale.Minimum"=w484, "XScale.Maximum"=w483) -> ()  [unwired: 2 in, 2 out]
                  }
                  frame 68 {
                    n439 = property on="Trigger histogram 68" class="XYGraph (strict)"("YScale.Maximum"=w488, "XScale.Minimum"=w487, "XScale.Maximum"=w486) -> ()  [unwired: 2 in, 2 out]
                  }
                  frame 69 {
                    n440 = property on="Trigger histogram 69" class="XYGraph (strict)"("YScale.Maximum"=w491, "XScale.Minimum"=w490, "XScale.Maximum"=w489) -> ()  [unwired: 2 in, 2 out]
                  }
                  frame 70 {
                    n441 = property on="Trigger histogram 70" class="XYGraph (strict)"("YScale.Maximum"=w494, "XScale.Minimum"=w493, "XScale.Maximum"=w492) -> ()  [unwired: 2 in, 2 out]
                  }
                  frame 71 {
                    n442 = property on="Trigger histogram 71" class="XYGraph (strict)"("YScale.Maximum"=w497, "XScale.Minimum"=w496, "XScale.Maximum"=w495) -> ()  [unwired: 2 in, 2 out]
                  }
                  frame 72 {
                    n443 = property on="Trigger histogram 72" class="XYGraph (strict)"("YScale.Maximum"=w500, "XScale.Minimum"=w499, "XScale.Maximum"=w498) -> ()  [unwired: 2 in, 2 out]
                  }
                  frame 73 {
                    n444 = property on="Trigger histogram 73" class="XYGraph (strict)"("YScale.Maximum"=w503, "XScale.Minimum"=w502, "XScale.Maximum"=w501) -> ()  [unwired: 2 in, 2 out]
                  }
                  frame 74 {
                    n445 = property on="Trigger histogram 74" class="XYGraph (strict)"("YScale.Maximum"=w506, "XScale.Minimum"=w505, "XScale.Maximum"=w504) -> ()  [unwired: 2 in, 2 out]
                  }
                  frame 75 {
                    n446 = property on="Trigger histogram 75" class="XYGraph (strict)"("YScale.Maximum"=w509, "XScale.Minimum"=w508, "XScale.Maximum"=w507) -> ()  [unwired: 2 in, 2 out]
                  }
                  frame 76 {
                    n447 = property on="Trigger histogram 76" class="XYGraph (strict)"("YScale.Maximum"=w512, "XScale.Minimum"=w511, "XScale.Maximum"=w510) -> ()  [unwired: 2 in, 2 out]
                  }
                  frame 77 {
                    n448 = property on="Trigger histogram 77" class="XYGraph (strict)"("YScale.Maximum"=w515, "XScale.Minimum"=w514, "XScale.Maximum"=w513) -> ()  [unwired: 2 in, 2 out]
                  }
                  frame 78 {
                    n449 = property on="Trigger histogram 78" class="XYGraph (strict)"("YScale.Maximum"=w518, "XScale.Minimum"=w517, "XScale.Maximum"=w516) -> ()  [unwired: 2 in, 2 out]
                  }
                  frame 79 {
                    n450 = property on="Trigger histogram 79" class="XYGraph (strict)"("YScale.Maximum"=w521, "XScale.Minimum"=w520, "XScale.Maximum"=w519) -> ()  [unwired: 2 in, 2 out]
                  }
                  frame 80 {
                    n451 = property on="Trigger histogram 80" class="XYGraph (strict)"("YScale.Maximum"=w524, "XScale.Minimum"=w523, "XScale.Maximum"=w522) -> ()  [unwired: 2 in, 2 out]
                  }
                  frame 81 {
                    n452 = property on="Trigger histogram 81" class="XYGraph (strict)"("YScale.Maximum"=w527, "XScale.Minimum"=w526, "XScale.Maximum"=w525) -> ()  [unwired: 2 in, 2 out]
                  }
                  frame 82 {
                    n453 = property on="Trigger histogram 82" class="XYGraph (strict)"("YScale.Maximum"=w530, "XScale.Minimum"=w529, "XScale.Maximum"=w528) -> ()  [unwired: 2 in, 2 out]
                  }
                  frame 83 {
                    n454 = property on="Trigger histogram 83" class="XYGraph (strict)"("YScale.Maximum"=w533, "XScale.Minimum"=w532, "XScale.Maximum"=w531) -> ()  [unwired: 2 in, 2 out]
                  }
                  frame 84 {
                    n455 = property on="Trigger histogram 84" class="XYGraph (strict)"("YScale.Maximum"=w536, "XScale.Minimum"=w535, "XScale.Maximum"=w534) -> ()  [unwired: 2 in, 2 out]
                  }
                  frame 85 {
                    n456 = property on="Trigger histogram 85" class="XYGraph (strict)"("YScale.Maximum"=w539, "XScale.Minimum"=w538, "XScale.Maximum"=w537) -> ()  [unwired: 2 in, 2 out]
                  }
                  frame 86 {
                    n457 = property on="Trigger histogram 86" class="XYGraph (strict)"("YScale.Maximum"=w542, "XScale.Minimum"=w541, "XScale.Maximum"=w540) -> ()  [unwired: 2 in, 2 out]
                  }
                  frame 87 {
                    n458 = property on="Trigger histogram 87" class="XYGraph (strict)"("YScale.Maximum"=w545, "XScale.Minimum"=w544, "XScale.Maximum"=w543) -> ()  [unwired: 2 in, 2 out]
                  }
                  frame 88 {
                    n459 = property on="Trigger histogram 88" class="XYGraph (strict)"("YScale.Maximum"=w548, "XScale.Minimum"=w547, "XScale.Maximum"=w546) -> ()  [unwired: 2 in, 2 out]
                  }
                  frame 89 {
                    n460 = property on="Trigger histogram 89" class="XYGraph (strict)"("YScale.Maximum"=w551, "XScale.Minimum"=w550, "XScale.Maximum"=w549) -> ()  [unwired: 2 in, 2 out]
                  }
                  frame 90 {
                    n461 = property on="Trigger histogram 90" class="XYGraph (strict)"("YScale.Maximum"=w554, "XScale.Minimum"=w553, "XScale.Maximum"=w552) -> ()  [unwired: 2 in, 2 out]
                  }
                  frame 91 {
                    n462 = property on="Trigger histogram 91" class="XYGraph (strict)"("YScale.Maximum"=w557, "XScale.Minimum"=w556, "XScale.Maximum"=w555) -> ()  [unwired: 2 in, 2 out]
                  }
                  frame 92 {
                    n463 = property on="Trigger histogram 92" class="XYGraph (strict)"("YScale.Maximum"=w560, "XScale.Minimum"=w559, "XScale.Maximum"=w558) -> ()  [unwired: 2 in, 2 out]
                  }
                  frame 93 {
                    n464 = property on="Trigger histogram 93" class="XYGraph (strict)"("YScale.Maximum"=w563, "XScale.Minimum"=w562, "XScale.Maximum"=w561) -> ()  [unwired: 2 in, 2 out]
                  }
                  frame 94 {
                    n465 = property on="Trigger histogram 94" class="XYGraph (strict)"("YScale.Maximum"=w566, "XScale.Minimum"=w565, "XScale.Maximum"=w564) -> ()  [unwired: 2 in, 2 out]
                  }
                  frame 95 {
                    n466 = property on="Trigger histogram 95" class="XYGraph (strict)"("YScale.Maximum"=w569, "XScale.Minimum"=w568, "XScale.Maximum"=w567) -> ()  [unwired: 2 in, 2 out]
                  }
                  frame 96 {
                    n467 = property on="Trigger histogram 96" class="XYGraph (strict)"("YScale.Maximum"=w572, "XScale.Minimum"=w571, "XScale.Maximum"=w570) -> ()  [unwired: 2 in, 2 out]
                  }
                  frame 97 {
                    n468 = property on="Trigger histogram 97" class="XYGraph (strict)"("YScale.Maximum"=w575, "XScale.Minimum"=w574, "XScale.Maximum"=w573) -> ()  [unwired: 2 in, 2 out]
                  }
                  frame 98 {
                    n469 = property on="Trigger histogram 98" class="XYGraph (strict)"("YScale.Maximum"=w578, "XScale.Minimum"=w577, "XScale.Maximum"=w576) -> ()  [unwired: 2 in, 2 out]
                  }
                  frame 99 {
                    n470 = property on="Trigger histogram 99" class="XYGraph (strict)"("YScale.Maximum"=w581, "XScale.Minimum"=w580, "XScale.Maximum"=w579) -> ()  [unwired: 2 in, 2 out]
                  }
                }
              }
            }
            event "Take image button": Mouse Down {
              w582 = FALSE
              n471 = event-data() -> ()  [unwired: 1 in, 7 out]
              n472 = flat-sequence {
                tunnel: [w584] -> w583
                tunnel: w583 -> [w594]
                frame #0 {
                  n473 = local read "ACQ full DATA file path"() -> (w590:path)
                  n474 = local read "Chip ID"() -> (w589:string)
                  n475 = Strip Path(path=w590) -> (stripped path=w587:path)  [unwired: 1 out]
                  n476 = Concatenate Strings(w589, "_ACQ_histograms.png" ("name or relative path")) -> (w585:string)
                  n477 = invoke class="VI" method="FP.Get Image"("image depth"=24 ("Image Depth")) -> ("image data"=w592:T3)  [unwired: 5 in, 5 out]
                  n478 = Build Path(base path=w587, name or relative path=w585) -> (appended path=w591:path)
                  n479 = call <vilib>:"Write PNG File.vi"("image data"=w592, "path to PNG file"=w591) -> ()  [unwired: 8 in, 2 out]
                  n480 = Concatenate Strings("Image saved\n", w585) -> (w584:string)
                }
                frame #1 {
                  n481 = call "MessageTimeOk.vi"("time (ms)"=2500, "missage"=w594) -> ()  [unwired: 4 in]
                }
              }
            }
          }
        }
      }
    }
  }
